vi "Process_data.vi"(3 "No of estimates output":i32=200, 4 "Measurement top level?":bool) -> (6 "Vel stat display":string[][](table), 7 "First Plot data Cluster":cluster{"X array":dbl[], "Y array":dbl[]}[](array[cluster]), 8 "Second Plot Data Cluster":cluster{"X array":dbl[], "Y array":dbl[]}[](array[cluster]))   [LabVIEW 2022 SP3]
uses:
  Controls/Inst_type.ctl
  Controls/Instrument_Array.ctl
  Controls/Post_Process.ctl
  Controls/User_Specific_mode.ctl
  Controls/Server_Comms.ctl
  <vilib>/Analysis/baseanly.llb/Mean (DBL).vi
  Globals/Meas_global.vi
  Globals/Dynamic_call_global.ph.vi
  CTA/CTA Calib Coeff Global.vi
  Globals/LDA_global.vi
  Globals/LDA_meas_global_1.vi
  Acquisition/PWA/PWAtasksGLOBAL.vi
  Globals/Trav_pos_global.vi
  Globals/Preference_global.vi
  <vilib>/Analysis/NI_AALBase.lvlib
panel:
  out "Extra Comments":string
  out "Over/Under string":string
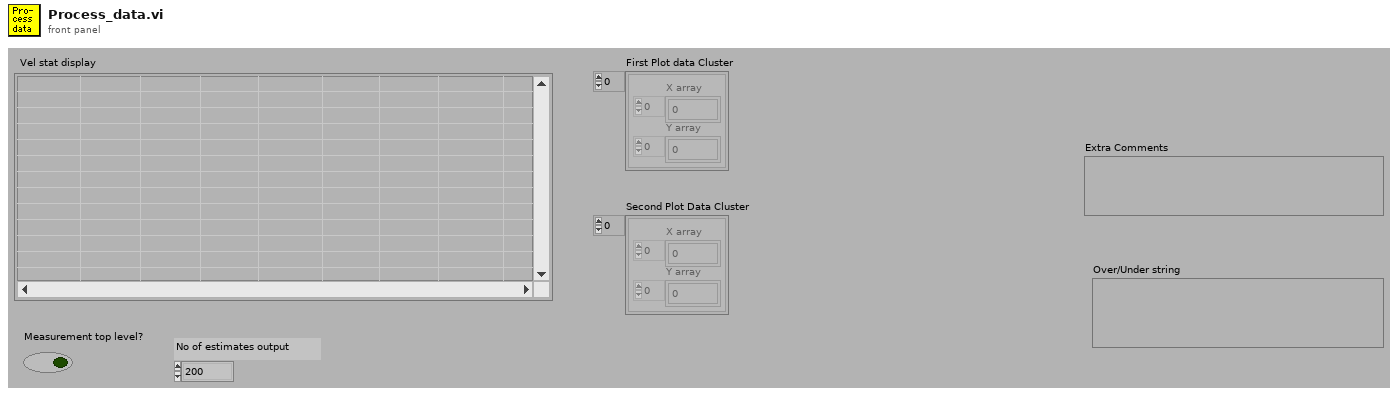
[diagram p1: front panel]
types:
  T1 = typedef "Inst_type.ctl" = enum16{"Raw voltage", "Raw with zero offsetting", "Propeller anemometer", "Pressure Transducer", "Pitot-static tube", "Hot wire", "Cross wire 1", "Cross wire 2", "Generic Linear", "Generic Polynomial", "Generic BackPoly", "Fast FID", "Thermocouple", "Cold wire", "Pulsed Wire", "LDA Vel", "LDA Tran time", "LDA Arr time", "Microphone"}
  T2 = typedef "Instrument_Array.ctl" = enum16{"PWA", "LDA", "Analogue"}
  T3 = enum32{"Invalid", "Standard", "Closed", "Hidden", "Minimized", "Maximized"}
  T4 = typedef "Post_Process.ctl" = enum16{"Take New Data", "Post Process Raw Data File"}
  T5 = typedef "User_Specific_mode.ctl" = enum16{"Check VI only", "Run VI"}
  T6 = enum16{"Save no data", "Save data in new files", "Save data in existing files"}
  T7 = typedef "Server_Comms.ctl" = enum16{"Do Not Link To Server", "Server Link Healthy"}
  T8 = typedef "Analysis_info_cluster.ctl" = cluster{"Colour":u32, "Inst type":T1, "Inst name":string, "Symbol":string, "Code name":string, "Extra Info":string, "Inst Array":T2, "U":dbl, "u^2":dbl, "u^3":dbl, "u^4":dbl, "Skew_u":dbl, "Kurt_u":dbl, "Sd Error in Mean":dbl, "% u'/U":dbl, "X":dbl, "Y":dbl, "Z":dbl, "Timescale integral Estimate":dbl, "Sd Error in Variance":dbl, "Calib File":path, "Calib Constants":dbl[], "Output Position":bool, "Stats":enum16{"None", "Basic", "Full"}, "Av Sampling Rate":dbl, "Av No of Samples":dbl, "Total Meas Time (s)":dbl, "OrigChName":string, "Max value":dbl, "Min value":dbl, "Req Sample Rate Hz":dbl, "Sync Delay Time (s)":dbl, "Ch No":i16, "Device":string, "Use Latest Calib":bool, "Port":string, "Metadata Ch Names":string[], "Metadata Ch Values":string[], "Label":string, "chState":T9, "Point Drift":dbl, "inputConfig":string}
  T9 = typedef "channelState.ctl" = enum32{"No Selection", "Solo", "Mute"}
  T10 = typedef "Time_Trace_Cluster.ctl" = cluster{"Weighting":dbl[], "Voltage":dbl[], "Eng Values":dbl[]}
  T11 = typedef "Calibration data.ctl" = cluster{"X cal.[]":dbl[], "Re cal.[]":dbl[], "a1[]":dbl[], "a2[]":dbl[], "a3[]":dbl[]}
  T12 = typedef "LDA_Channel.ctl" = cluster{"Wavelength (nm)":dbl, "Vel Comp":string, "Max Velocity":dbl, "Min Velocity":dbl, "Max Record length":u16, "Signal gain (dB)":i16, "High voltage":i16, "Optics Conversion Factor":dbl, "Min Record length":u16, "Multiply Velocity by -1":bool, "Signal to Noise Ratio":string, "Validation Ratio":string, "Probe":string, "Laser":string, "BSA":string, "Lense":string, "Beam Separation (mm)":dbl, "Focal Length (mm)":dbl, "COLOUR":u32, "BSA IP":string, "Velocity Range (m/s)":dbl, "Centre Velocity (m/s)":dbl, "Unshifted mW":dbl, "Shifted mW":dbl, "Bandwidth Hz":dbl, "Req Sampling Rate Hz":dbl, "Ch":i32, "CenterFreq Hz":dbl, "Laser IP":string, "Sync Delay (s)":dbl}
  T13 = typedef "PWA_Data.ctl" = enum16{"No PWA Data", "One Ch PWA"}
  T14 = typedef "Resample mode.ctl" = cluster{"Mode":enum16{"Index", "Interpolate"}, "Index":dbl[]}
  T15 = typedef "Shift_Cluster.ctl" = cluster{"Stats":dbl[], "Spectra_Auto":dbl[], "Histogram":dbl[], "Hist Max":dbl, "Hist Min":dbl, "No of Samples":i32, "No in plume":i32, "Weight sum":dbl, "No Of Hist bins":i32, "TimeTrace Max":dbl, "Time Trace Min":dbl, "Trace St Deviation":dbl}
  T16 = typedef "XY_Plot_Cluster.ctl" = cluster{"First Name":string, "Second Name":string, "X axis name":string, "Y axis name":string, "X array":dbl[], "Y array":dbl[], "Weighting":dbl[]}
  T17 = typedef "Traverse_cluster.ctl" = cluster{"Start X":sgl, "Start Y":sgl, "Start Z":sgl, "End X":sgl, "End Y":sgl, "End Z":sgl, "nPoints":i32, "Spacing":T18, "Filename":path, "Tunnel Speed":dbl, "Averaging time (mins)":dbl, "Extra Commands":string, "Carrier_1 Q (l/min)":dbl, "Carrier_2 Q (l/min)":dbl, "Trace Gas Concentration (%)":dbl, "Specific Arguments":string, "Comments":string, "Row No":i32, "Row Type Selector":T19, "EstCompl":string, "Row Duration (mins)":dbl, "nValidPoints":i32, "Meas Setup File":string}
  T18 = typedef "Spacing.ctl" = enum16{"Linear", "Log", "Gauss", "Specified", "N/A"}
  T19 = typedef "Multi_run_mode.ctl" = enum16{"Move Traverse Only", "Set Tunnel Speed Only", "Set Source Only", "Set Measurement Conditions", "Single Measurement", "Vertical Profile", "Lateral Profile", "Longitudinal Profile", "Multi-Axis Profile", "Explore Volume", "Auto Calibrate", "Meas Fast FID Bkgnd", "Check Beam Power", "Scanning Valve Measurement", "Run VI Named:", "Set ADAM Ch", "Wait (minutes)", "Send Message", "Synchronize With:", "Fall Back to this Row", "Turn Off Row Repeating", "Traverse 3D Volume", "Blank Row", "Jump to Fall Back Row"}
  T20 = typedef "Cross_Moments_Shift_Cluster.ctl" = cluster{"Stats":dbl[], "Resampled No of Samples":i32, "Resampled delta T":dbl, "Cross Correlation":dbl[]}
  T21 = typedef "Correlation_cluster1.ctl" = cluster{"U inst":string, "uw":dbl, "u^2w":dbl, "uw^2":dbl, "uw/u'w'":dbl, "W inst":string, "uw^3":dbl, "u^3w":dbl, "u^2w^2":dbl, "Index U":i32, "Index W":i32, "Error info":string[], "Paired Sampling Rate (Hz)":dbl, "u^2 Paired":dbl, "w^2 Paired":dbl, "Time Window (ms)":dbl}
  T22 = typedef "Graph_Type.ctl" = enum16{"Show no graph", "Voltage trace", "Velocity trace", "Vel histogram", "Spectrum", "f.E(f) v Log f", "Auto-Corr"}
  T23 = cluster{"Plot 1":u16, "Plot 2":u16, "Save graph":u16, "Plot Type":T22}
  T24 = cluster{"Plot 1":u16, "Plot 2":u16, "Save graph":u16, "Plot Type":T22}[]
  T25 = typedef "Data for Inst Type.ctl" = enum16{"Eng Values", "Voltage"}
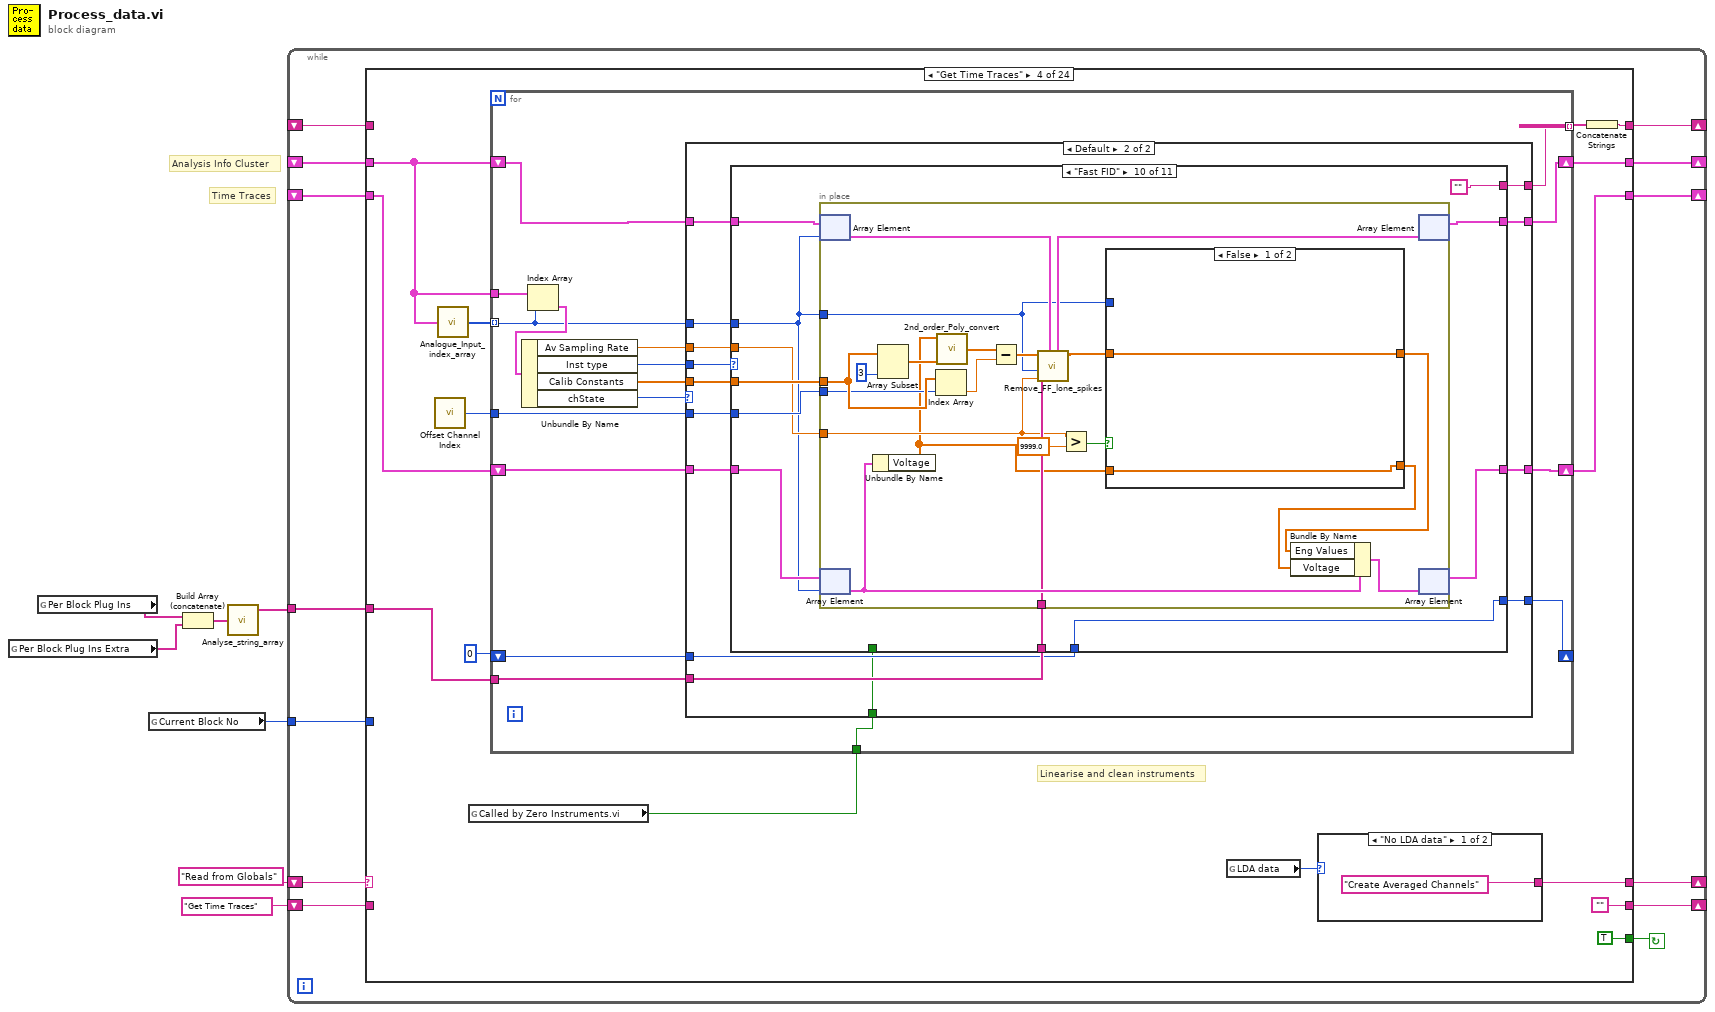
[diagram p0: block diagram]
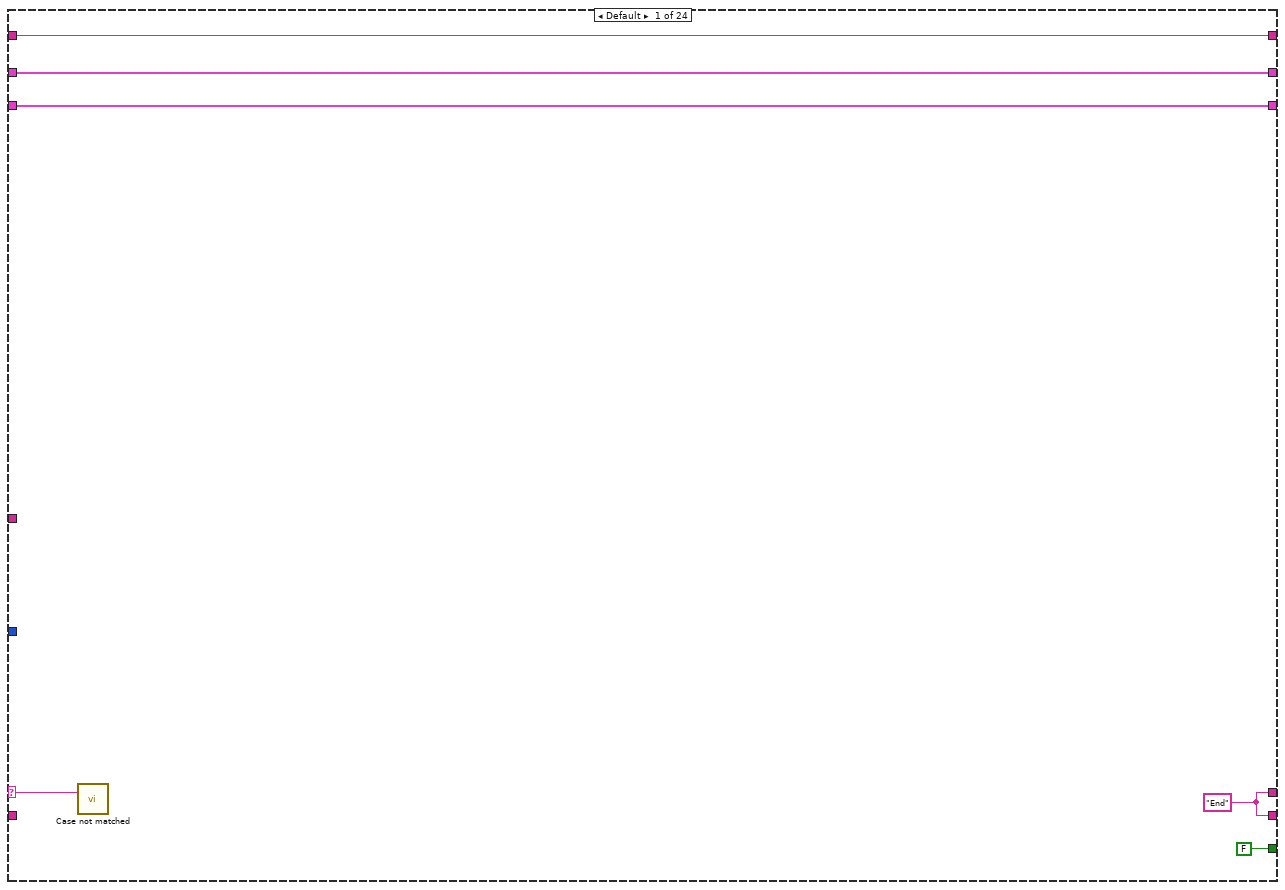
[diagram p2: hidden frame]
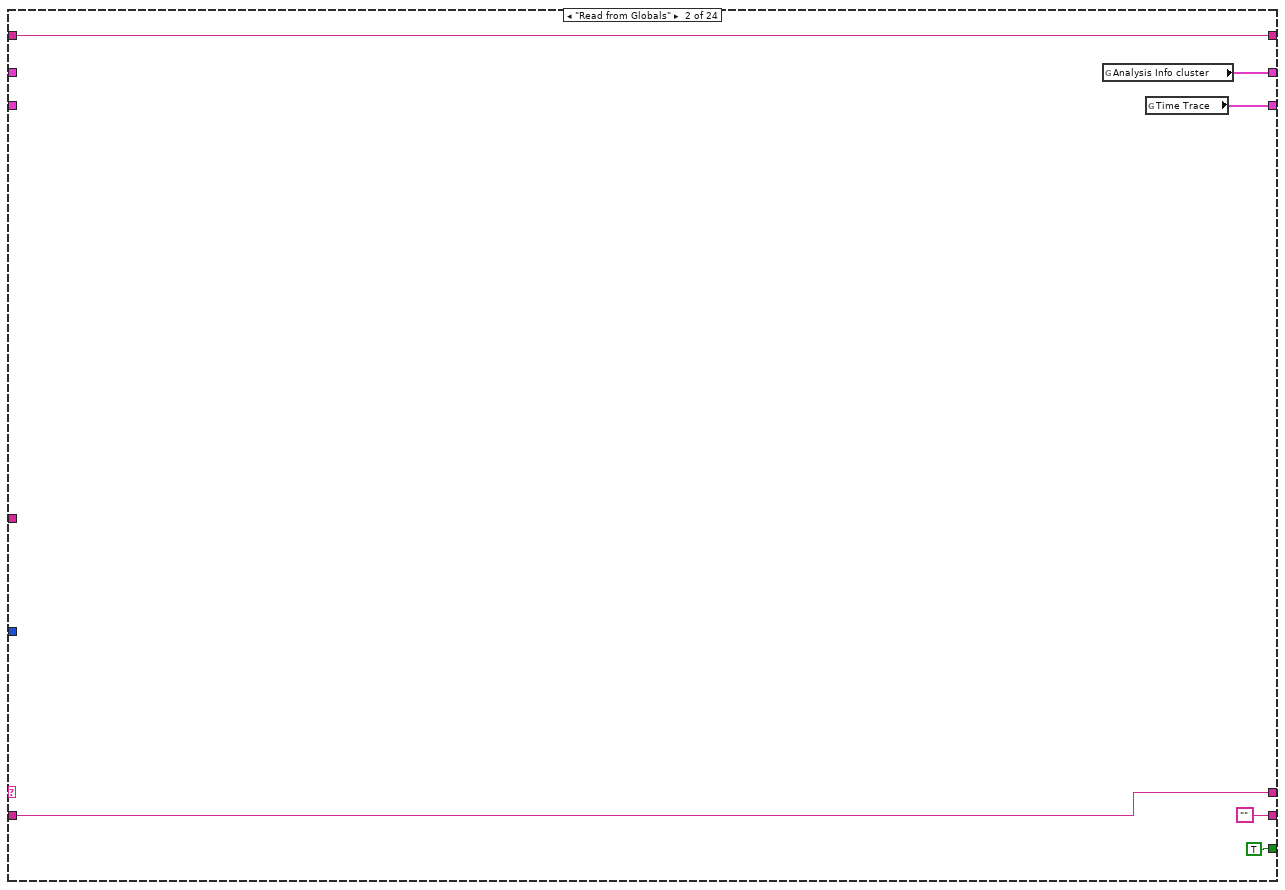
[diagram p3: hidden frame]
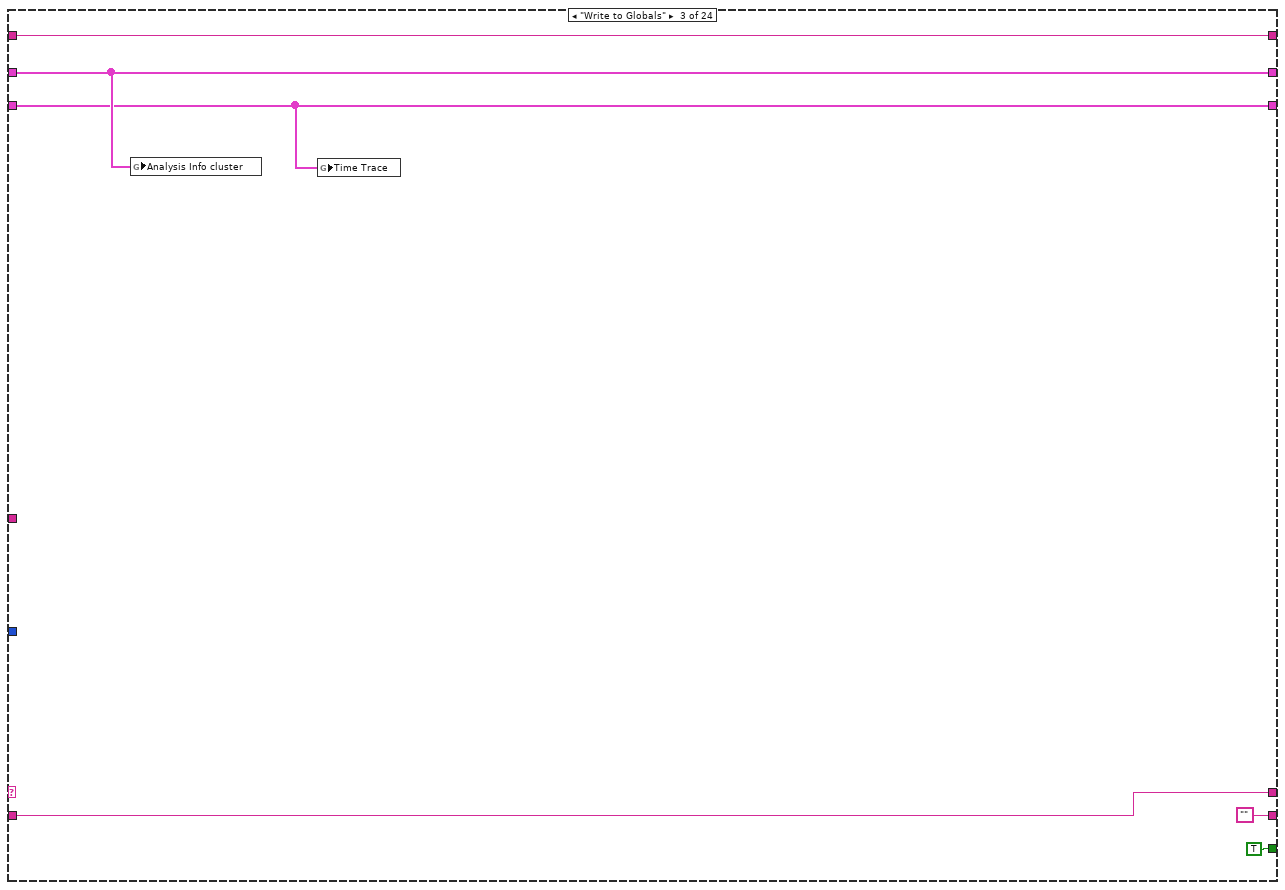
[diagram p4: hidden frame]
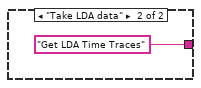
[diagram p5: hidden frame]
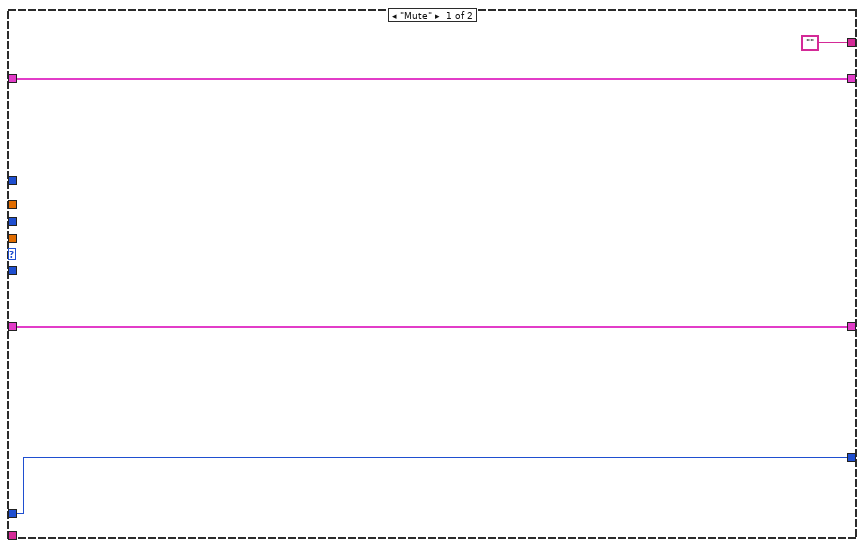
[diagram p6: hidden frame]
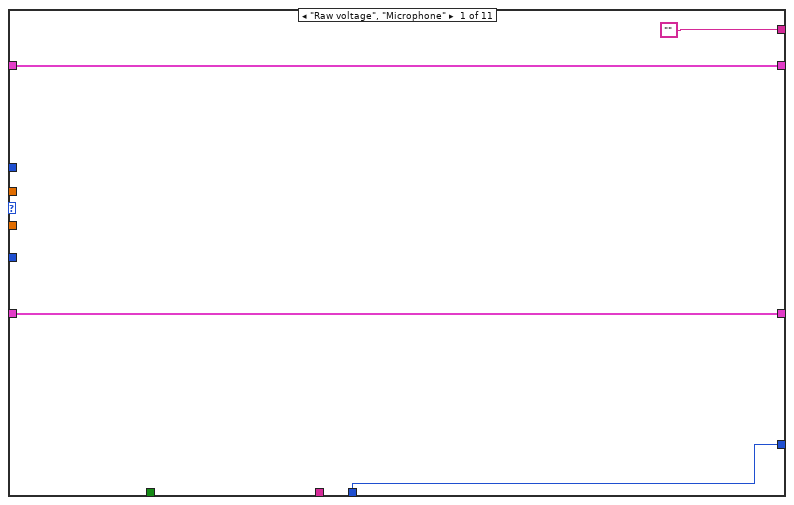
[diagram p7: hidden frame]
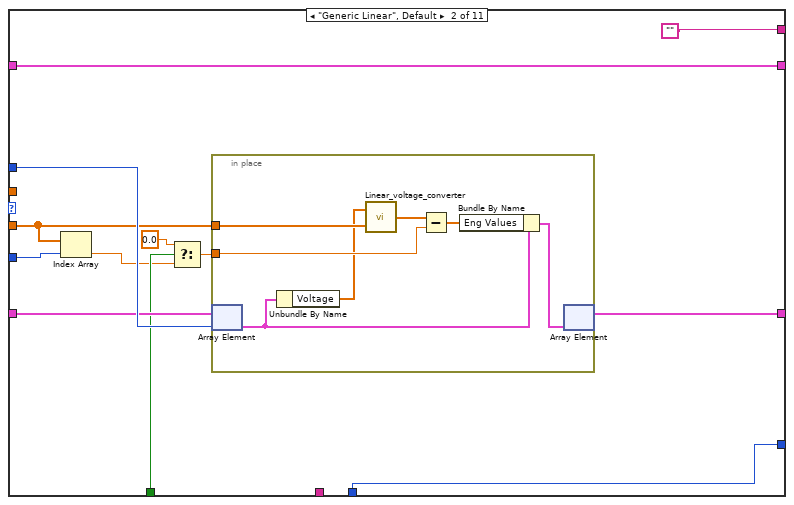
[diagram p8: hidden frame]
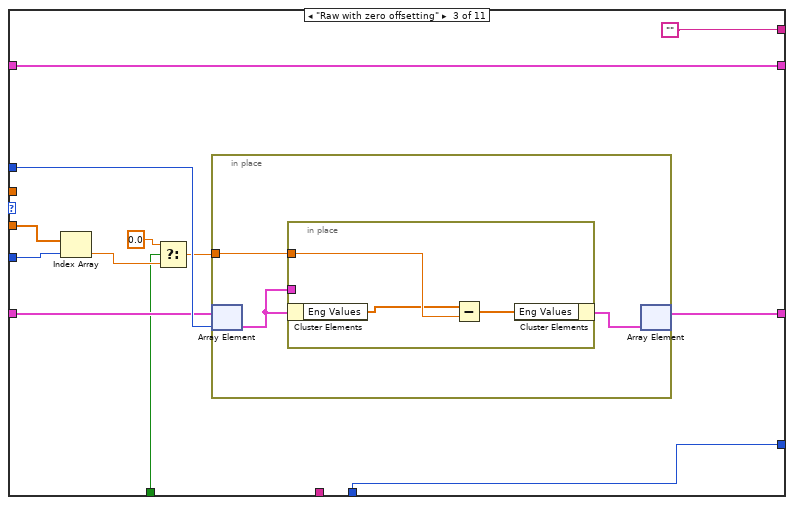
[diagram p9: hidden frame]
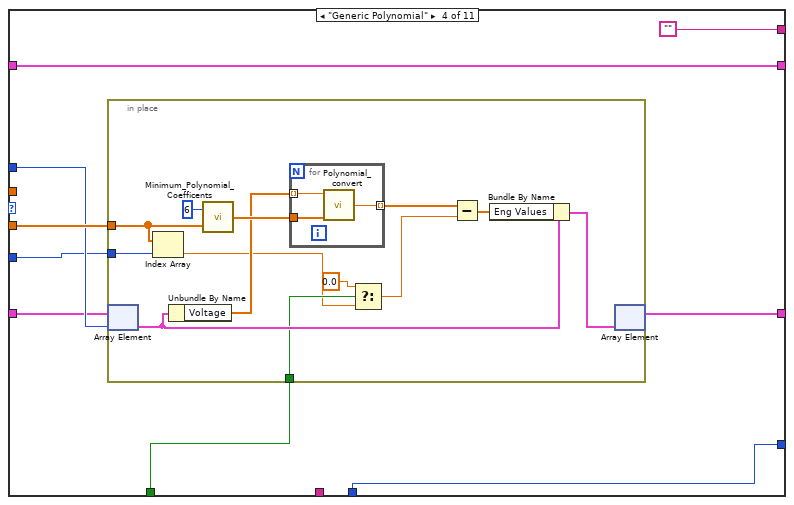
[diagram p10: hidden frame]
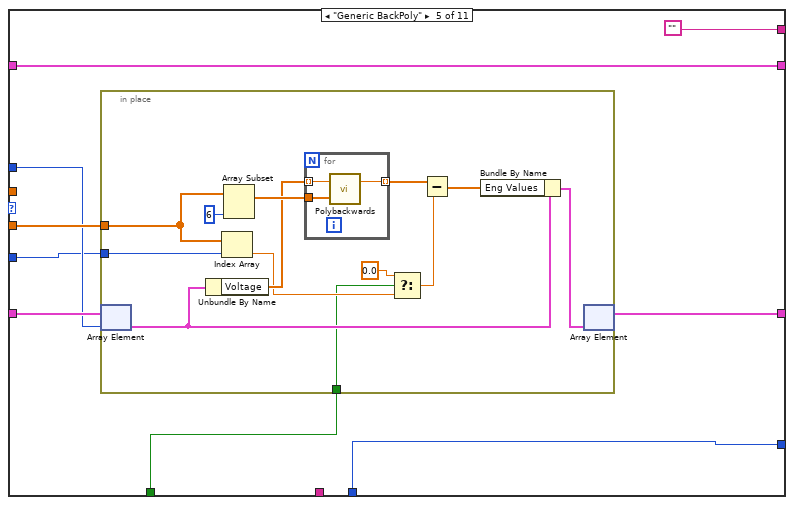
[diagram p11: hidden frame]
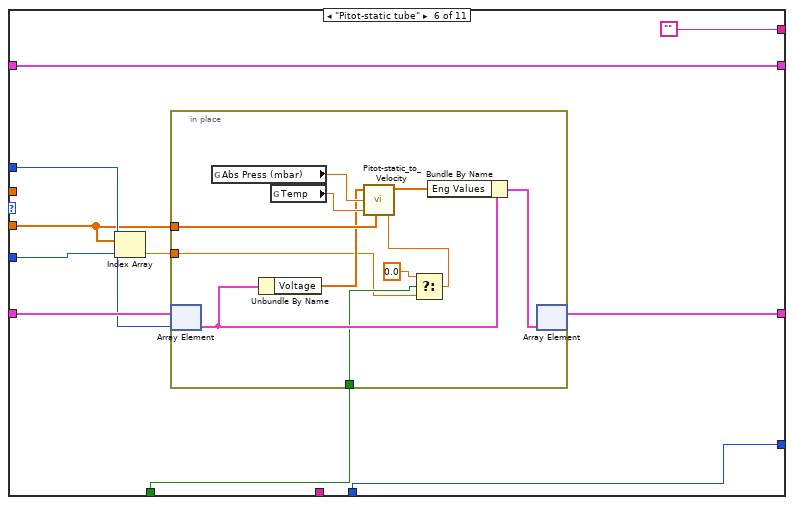
[diagram p12: hidden frame]
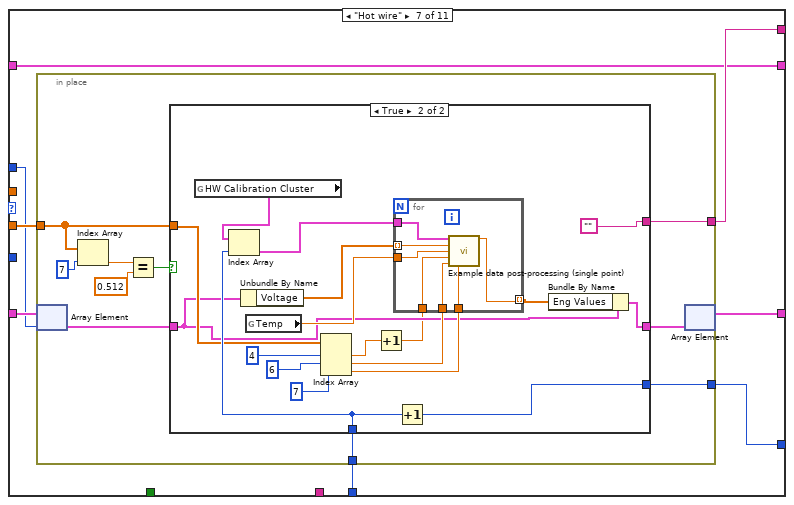
[diagram p13: hidden frame]
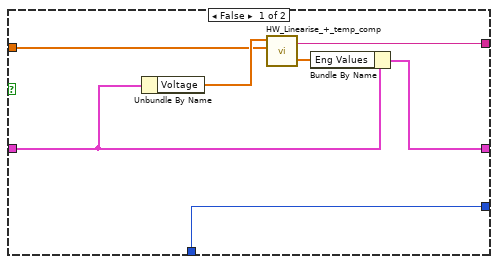
[diagram p14: hidden frame]
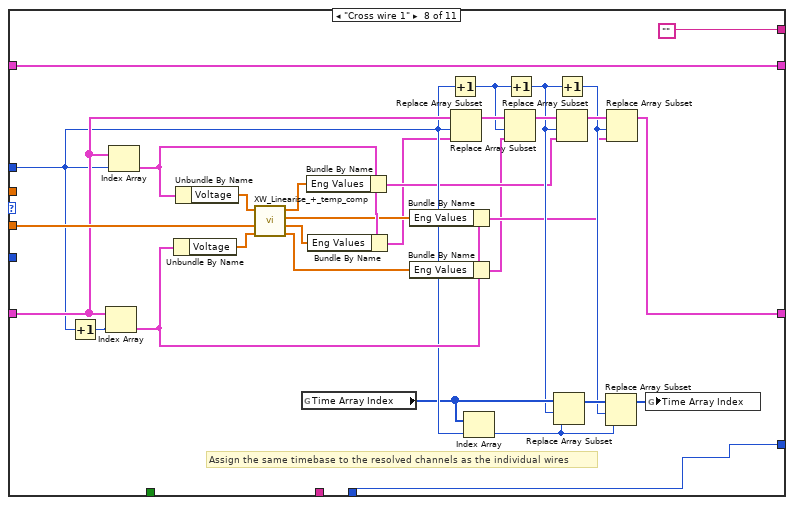
[diagram p15: hidden frame]
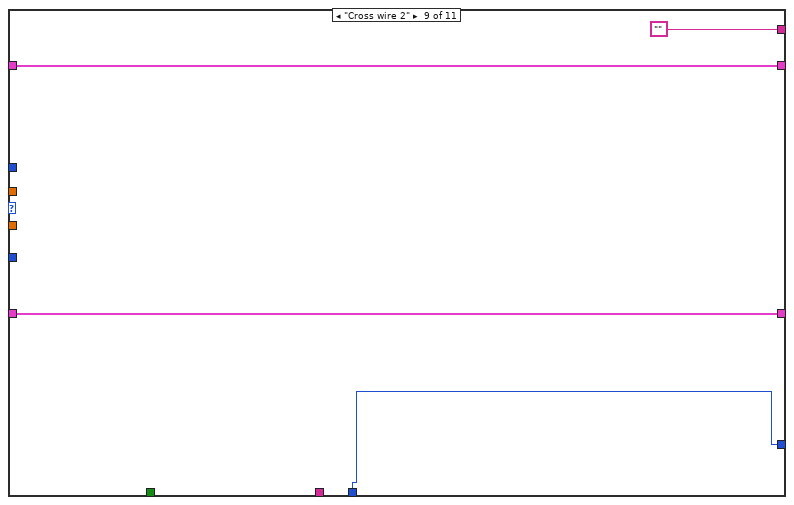
[diagram p16: hidden frame]
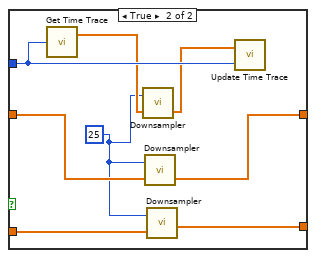
[diagram p17: hidden frame]
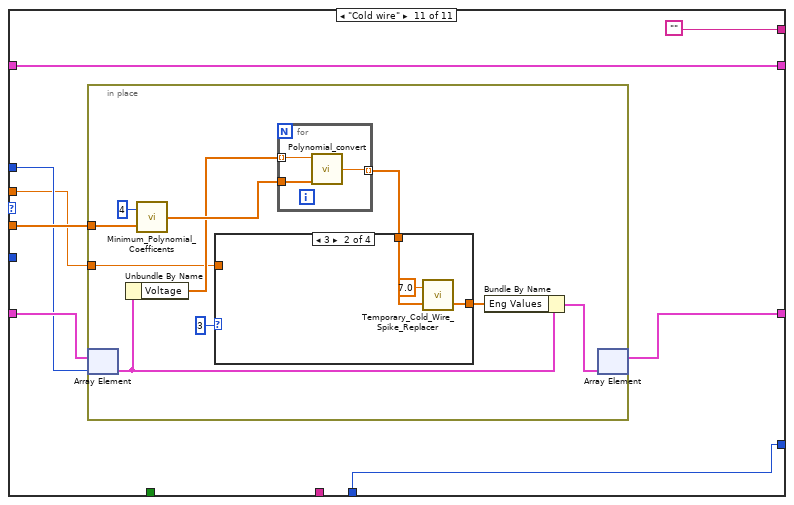
[diagram p18: hidden frame]
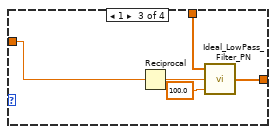
[diagram p20: hidden frame]
diagram:
  # "Time Traces"
  # "Analysis Info Cluster"
  n1 = global read "Dynamic_call_global.ph.vi" "Per Block Plug Ins Extra"() -> (w4:string[])
  n2 = global read "Dynamic_call_global.ph.vi" "Per Block Plug Ins"() -> (w3:string[])
  n3 = global read "Meas_global.vi" "Current Block No"() -> (w6:i32)
  n4 = Build Array (concatenate)(w3, w4) -> (w2:string[])
  n5 = call "Analyse_string_array.vi"("String array"=w2) -> ("Unique strings"=w1:string[])  [unwired: 2 out]
  n6 = while {
    shift-right: [w19] -> _
    shift-left: "Read from Globals" -> [w20]
    shift-right: [w17] -> _
    shift-left: _ -> [w18]
    shift-right: [w13] -> _
    shift-left: _ -> [w12]
    shift-right: [w16] -> _
    shift-left: _ -> [w14]
    tunnel: w6 -> [w11]
    shift-right: [w9] -> _
    shift-left: "Get Time Traces" -> [w10]
    tunnel: w1 -> [w8]
    stop <- w15 continue-if-true
    n7 = case shown="\"Get Time Traces\"" w20 {
      selector: w20 -> [w26 _ _ _ _ _ _ _ _ _ _ _ _ _ _ _ _ _ _ _ _ _ _ _]
      tunnel: [w21 w29 w37 w50 w363 "LDA_Angular_Alignment_Tweak" w507 "Any Pre Analysis Plugins?" w672 "Read from Globals" "Add Extra Data Channels" "Min Max Limiter" "Analysis of Time Traces" "Vel Stats Display" w920 "Write to Globals" "Write to Globals" w1162 w1174 "Output Cross moments" "Create Plot Clusters" "Seeder Control?" "Control Seeding level" "End"] -> w19
      tunnel: w12 -> [w23 _ w34 w44 w374 w442 w506 w607 w674 w690 w719 w821 w885 w912 w923 w1012 w1063 w1160 w1179 w1337 w1387 w1418 w1520 w1536]
      tunnel: w18 -> [w22 _ w33 w49 w377 w441 w523 w610 w673 w689 w718 w822 w888 w911 w922 w1013 w1067 w1164 w1176 w1336 w1386 w1420 w1519 w1534]
      tunnel: [w22 w31 w33 w48 w376 w441 w522 w605 w673 w689 w718 w823 w887 w911 w922 w1013 w1067 w1164 w1177 w1336 w1386 w1420 w1519 w1534] -> w17
      tunnel: [w24 w30 w38 w47 w378 w443 w521 w613 w675 w691 w720 w820 w886 w916 w924 w1011 w1068 w1165 w1181 w1354 w1388 w1425 w1521 w1535] -> w16
      tunnel: [FALSE TRUE TRUE TRUE TRUE TRUE TRUE TRUE TRUE TRUE TRUE TRUE TRUE TRUE TRUE TRUE TRUE TRUE w1173 TRUE TRUE w1426 w1531 FALSE] -> w15
      tunnel: w14 -> [w24 w30 w38 _ w379 w443 w521 w613 w675 w691 w720 w820 w886 w917 w924 w1011 w1068 w1165 w1180 w1354 w1388 w1425 w1521 w1535]
      tunnel: [w23 w32 w34 w43 w375 w442 w506 w607 w674 w690 w719 w821 w885 w905 w923 w1012 w1064 w1160 w1178 w1337 w1387 w1418 w1520 w1536] -> w13
      tunnel: w11 -> [_ _ _ _ w373 _ _ _ _ _ w715 _ _ _ _ _ _ _ w1175 _ _ _ _ _]
      tunnel: w10 -> [_ w29 w37 _ _ _ w514 _ _ _ _ _ _ _ _ _ _ _ _ _ _ _ _ _]
      tunnel: [w21 "" "" "" "" "1" w511 "" w671 "Add PWA Data" "" "" "" "" "" "Per Block Plug ins" "Per Block Plug ins" w1161 w1172 "" "" "" "" ""] -> w9
      tunnel: w8 -> [_ _ _ w41 _ _ _ _ _ _ _ _ _ _ _ _ _ w1159 _ _ _ _ _ _]
      frame Default {
        w21 = "End"
        n8 = call "Case not matched.vi"("Case Name not Matched"=w26) -> ()
      }
      frame "Read from Globals" {
        n9 = global read "Meas_global.vi" "Analysis Info cluster"() -> (w32:T8[])
        n10 = global read "Meas_global.vi" "Time Trace"() -> (w31:T10[])
      }
      frame "Write to Globals" {
        n11 = global write "Meas_global.vi" "Analysis Info cluster"(w34) -> ()
        n12 = global write "Meas_global.vi" "Time Trace"(w33) -> ()
      }
      frame "Get Time Traces" {
        # "Linearise and clean instruments"
        n13 = call "Offset Channel Index.vi"() -> ("index"=w42:i32)
        n14 = call "Analogue_Input_index_array.vi"("Analysis Info cluster"=w44) -> ("Array"=w53:i32[])
        n15 = global read "Meas_global.vi" "Called by Zero Instruments.vi"() -> (w39:bool)
        n16 = for {
          shift-right: [w69] -> w48
          shift-left: w49 -> [w70]
          tunnel: w44 -> [w72]
          tunnel: w53 -> [w66] mode=indexing
          tunnel: [w64] -> w52 mode=indexing
          shift-right: [w62] -> w43
          shift-left: w44 -> [w63]
          tunnel: w42 -> [w61]
          tunnel: w41 -> [w60]
          shift-right: [w58] -> _
          shift-left: 0 -> [w59]
          tunnel: w39 -> [w57]
          n17 = Index Array(array=w72, index=w66) -> (element=w71:T8)
          n18 = Unbundle By Name(w71) -> ("Av Sampling Rate"=w65:dbl, "Inst type"=w68:T1, "Calib Constants"=w67:dbl[], "chState"=w56:T9)
          n19 = case shown="Default" w56 {
            tunnel: w70 -> [w74 w90]
            tunnel: [w74 w89] -> w69
            tunnel: w68 -> [_ w88]
            tunnel: w67 -> [_ w87]
            tunnel: w66 -> [_ w86]
            tunnel: w65 -> [_ w85]
            tunnel: ["" w84] -> w64
            tunnel: w63 -> [w76 w83]
            tunnel: [w76 w82] -> w62
            tunnel: w61 -> [_ w81]
            tunnel: w60 -> [_ w80]
            tunnel: w59 -> [w73 w79]
            tunnel: [w73 w78] -> w58
            tunnel: w57 -> [_ w77]
            frame "Mute" {
            }
            frame Default {
              n20 = case shown="\"Fast FID\"" w88 {
                tunnel: w87 -> [_ w103 w122 w140 w165 w188 w210 w282 _ w297 w335]
                tunnel: w86 -> [_ w106 w125 w139 w163 w190 w207 w264 _ w288 w332]
                tunnel: w90 -> [w92 w105 w124 w138 w164 w191 w209 w276 w286 w296 w334]
                tunnel: [w92 w104 w123 w137 w162 w189 w208 w274 w286 w295 w333] -> w89
                tunnel: w81 -> [_ w102 w121 w136 w161 w187 _ _ _ w294 _]
                tunnel: w85 -> [_ _ _ _ _ _ _ _ _ w293 w331]
                tunnel: ["" "" "" "" "" "" w206 "" "" "" ""] -> w84
                tunnel: w83 -> [w93 w100 w119 w134 w159 w184 w205 w270 w284 w291 w329]
                tunnel: [w93 w100 w119 w134 w159 w184 w205 w270 w284 w290 w329] -> w82
                tunnel: w80 -> [_ _ _ _ _ _ _ _ _ w289 _]
                tunnel: w79 -> [w91 w99 w118 w133 w158 w183 w204 w253 w283 w287 w328]
                tunnel: [w91 w99 w118 w133 w158 w183 w203 w253 w283 w287 w328] -> w78
                tunnel: w77 -> [_ w98 w115 w132 w157 w182 _ _ _ _ _]
                frame "Raw voltage", "Microphone" {
                }
                frame "Generic Linear", Default {
                  n21 = Index Array(array=w103, index=w102) -> (element=w97:dbl)
                  n22 = Select(t=0.0, s=w98, f=w97) -> (s? t:f=w95:dbl)
                  n23 = in-place {
                    in-place-border: w103 -> [w113]
                    in-place-border: w95 -> [w109]
                    n24 = in-place-array #1(w105, w106) -> (w108:T10)
                    n25 = Unbundle By Name(w108) -> ("Voltage"=w107:dbl[])
                    n26 = call "Linear_voltage_converter.vi"("Caib const A,B"=w113, "Voltage array"=w107) -> ("Converted array"=w111:dbl[])
                    n27 = Subtract(x=w111, y=w109) -> (x-y=w110:dbl[])
                    n28 = Bundle By Name(cluster=w108, "Eng Values"=w110) -> (w112:T10)
                    n29 = in-place-array #1(w112) -> (w104:T10[])  [unwired: 1 out]
                  }
                }
                frame "Raw with zero offsetting" {
                  n30 = Index Array(array=w122, index=w121) -> (element=w116:dbl)
                  n31 = Select(t=0.0, s=w115, f=w116) -> (s? t:f=w114:dbl)
                  n32 = in-place {
                    in-place-border: w114 -> [w128]
                    n33 = in-place-array #2(w124, w125) -> (w127:T10)
                    n34 = in-place {
                      in-place-border: w128 -> [w131]
                      in-place-border: w127 -> [_]
                      n35 = in-place-cluster #3(w127) -> ("Eng Values"=w129:dbl[])
                      n36 = Subtract(x=w129, y=w131) -> (x-y=w130:dbl[])
                      n37 = in-place-cluster #3("Eng Values"=w130) -> (w126:T10)
                    }
                    n38 = in-place-array #2(w126) -> (w123:T10[])  [unwired: 1 out]
                  }
                }
                frame "Generic Polynomial" {
                  n39 = in-place {
                    in-place-border: w140 -> [w148]
                    in-place-border: w136 -> [w147]
                    in-place-border: w132 -> [w143]
                    n40 = in-place-array #4(w138, w139) -> (w146:T10)
                    n41 = Index Array(array=w148, index=w147) -> (element=w142:dbl)
                    n42 = Unbundle By Name(w146) -> ("Voltage"=w145:dbl[])
                    n43 = call "Minimum_Polynomial_Coefficents.vi"("Calib consts"=w148, "Max Length"=6) -> ("Coefficients"=w152:dbl[])
                    n44 = for {
                      tunnel: w152 -> [w156]
                      tunnel: w145 -> [w155] mode=indexing
                      tunnel: [w154] -> w150 mode=indexing
                      n45 = call "Polynomial_convert.vi"("Calib constants"=w156, "Voltage"=w155) -> ("Eng Values"=w154:dbl)  [unwired: 4 out]
                    }
                    n46 = Select(t=0.0, s=w143, f=w142) -> (s? t:f=w141:dbl)
                    n47 = Subtract(x=w150, y=w141) -> (x-y=w149:dbl[])
                    n48 = Bundle By Name(cluster=w146, "Eng Values"=w149) -> (w151:T10)
                    n49 = in-place-array #4(w151) -> (w137:T10[])  [unwired: 1 out]
                  }
                }
                frame "Generic BackPoly" {
                  n50 = in-place {
                    in-place-border: w165 -> [w175]
                    in-place-border: w161 -> [w174]
                    in-place-border: w157 -> [w166]
                    n51 = in-place-array #5(w164, w163) -> (w171:T10)
                    n52 = Unbundle By Name(w171) -> ("Voltage"=w170:dbl[])
                    n53 = Index Array(array=w175, index=w174) -> (element=w168:dbl)
                    n54 = Array Subset(array=w175, length=6) -> (w178:dbl[])  [unwired: 1 in]
                    n55 = for {
                      tunnel: w178 -> [w181]
                      tunnel: w170 -> [w180] mode=indexing
                      tunnel: [w179] -> w173 mode=indexing
                      n56 = call "Polybackwards.vi"("Coefficients"=w181, "Y input"=w180) -> ("X output"=w179:dbl)  [unwired: 1 out]
                    }
                    n57 = Select(t=0.0, s=w166, f=w168) -> (s? t:f=w167:dbl)
                    n58 = Subtract(x=w173, y=w167) -> (x-y=w172:dbl[])
                    n59 = Bundle By Name(cluster=w171, "Eng Values"=w172) -> (w176:T10)
                    n60 = in-place-array #5(w176) -> (w162:T10[])  [unwired: 1 out]
                  }
                }
                frame "Pitot-static tube" {
                  n61 = Index Array(array=w188, index=w187) -> (element=w186:dbl)
                  n62 = in-place {
                    in-place-border: w188 -> [w202]
                    in-place-border: w186 -> [w193]
                    in-place-border: w182 -> [w194]
                    n63 = in-place-array #6(w191, w190) -> (w197:T10)
                    n64 = global read "Meas_global.vi" "Abs Press (mbar)"() -> (w201:dbl)
                    n65 = Unbundle By Name(w197) -> ("Voltage"=w196:dbl[])
                    n66 = global read "Meas_global.vi" "Temp"() -> (w198:dbl)
                    n67 = Select(t=0.0, s=w194, f=w193) -> (s? t:f=w192:dbl)
                    n68 = call "Pitot-static_to_Velocity.vi"("Pressure Trans voltage"=w196, "Atmos Press mbar  (1000)"=w201, "Temp  C  (20)"=w198, "Pressure Trans Calib const"=w202, "Mano Zero"=w192) -> ("Velocity (m/s)"=w200:dbl[])  [unwired: 1 in, 2 out]
                    n69 = Bundle By Name(cluster=w197, "Eng Values"=w200) -> (w199:T10)
                    n70 = in-place-array #6(w199) -> (w189:T10[])  [unwired: 1 out]
                  }
                }
                frame "Hot wire" {
                  n71 = in-place {
                    in-place-border: w210 -> [w216]
                    in-place-border: [w218] -> w206
                    in-place-border: w204 -> [w215]
                    in-place-border: [w214] -> w203
                    n72 = in-place-array #7(w209, w207) -> (w219:T10)
                    n73 = Index Array(array=w216, index=7) -> (element=w213:dbl)
                    n74 = Equal?(x=w213, y=0.512) -> (x = y?=w212:bool)
                    n75 = case shown="True" w212 {
                      tunnel: [w226 w230] -> w220
                      tunnel: w219 -> [w225 w231]
                      tunnel: [w224 ""] -> w218
                      tunnel: w216 -> [w222 w239]
                      tunnel: w215 -> [w221 w244]
                      tunnel: [w221 w243] -> w214
                      frame False {
                        n76 = Unbundle By Name(w225) -> ("Voltage"=w223:dbl[])
                        n77 = call "HW_Linearise_+_temp_comp.vi"("Caib const"=w222, "HW voltage"=w223) -> ("Velocity"=w227:dbl[], "Error string"=w224:string)  [unwired: 4 in]
                        n78 = Bundle By Name(cluster=w225, "Eng Values"=w227) -> (w226:T10)
                      }
                      frame True {
                        n79 = global read "CTA Calib Coeff Global.vi" "HW Calibration Cluster"() -> (w245:T11[])
                        n80 = Index Array(array=w245, index=w244) -> (element=w242:T11)
                        n81 = Unbundle By Name(w231) -> ("Voltage"=w241:dbl[])
                        n82 = global read "Meas_global.vi" "Temp"() -> (w240:dbl)
                        n83 = Index Array(array=w239, index #1=4 ("index"), index #2=6 ("index"), index #3=7 ("index")) -> (element #1=w238:dbl, element #2=w237:dbl, element #3=w236:dbl)
                        n84 = Increment(x=w238) -> (x+1=w228:dbl)
                        n85 = for {
                          tunnel: w242 -> [w252]
                          tunnel: w241 -> [w251] mode=indexing
                          tunnel: w240 -> [w250]
                          tunnel: w228 -> [w249]
                          tunnel: w237 -> [w248]
                          tunnel: w236 -> [w247]
                          tunnel: [w246] -> w232 mode=indexing
                          n86 = call "Example data post-processing (single point).vi"("Calibration data"=w252, "V_out (V)"=w251, "Ta (°C)"=w250, "Overheat ratio (Rw / R0)"=w249, "Gain"=w248, "Offset (V)"=w247) -> ("U (m/s)"=w246:dbl)  [unwired: 9 in]
                        }
                        n87 = Increment(x=w244) -> (x+1=w243:i32)
                        n88 = Bundle By Name(cluster=w231, "Eng Values"=w232) -> (w230:T10)
                      }
                    }
                    n89 = in-place-array #7(w220) -> (w208:T10[])  [unwired: 1 out]
                  }
                }
                frame "Cross wire 1" {
                  # "Assign the same timebase to the resolved channels as the individual wires"
                  n90 = Increment(x=w264) -> (x+1=w279:i32)
                  n91 = Index Array(array=w276, index=w279) -> (element=w277:T10)
                  n92 = Index Array(array=w276, index=w264) -> (element=w278:T10)
                  n93 = Unbundle By Name(w277) -> ("Voltage"=w281:dbl[])
                  n94 = Unbundle By Name(w278) -> ("Voltage"=w280:dbl[])
                  n95 = call "XW_Linearise_+_temp_comp.vi"("XW2 voltage"=w281, "Calib const"=w282, "XW1 voltage"=w280) -> ("V"=w265:dbl[], "U"=w266:dbl[], "U2"=w267:dbl[], "U1"=w268:dbl[])  [unwired: 5 in]
                  n96 = global read "Meas_global.vi" "Time Array Index"() -> (w263:i32[])
                  n97 = Bundle By Name(cluster=w278, "Eng Values"=w268) -> (w257:T10)
                  n98 = Bundle By Name(cluster=w278, "Eng Values"=w266) -> (w256:T10)
                  n99 = Bundle By Name(cluster=w277, "Eng Values"=w267) -> (w255:T10)
                  n100 = Bundle By Name(cluster=w277, "Eng Values"=w265) -> (w254:T10)
                  n101 = Increment(x=w264) -> (x+1=w269:i32)
                  n102 = Replace Array Subset(array=w276, new element=w256, index=w264) -> (w275:T10[])
                  n103 = Index Array(array=w263, index=w264) -> (element=w259:i32)
                  n104 = Replace Array Subset(array=w275, new element=w254, index=w269) -> (w273:T10[])
                  n105 = Increment(x=w269) -> (x+1=w262:i32)
                  n106 = Replace Array Subset(array=w263, new element=w259, index=w262) -> (w261:i32[])
                  n107 = Increment(x=w262) -> (x+1=w260:i32)
                  n108 = Replace Array Subset(array=w273, new element=w257, index=w262) -> (w272:T10[])
                  n109 = Replace Array Subset(array=w261, new element=w259, index=w260) -> (w258:i32[])
                  n110 = Replace Array Subset(array=w272, new element=w255, index=w260) -> (w274:T10[])
                  n111 = global write "Meas_global.vi" "Time Array Index"(w258) -> ()
                }
                frame "Cross wire 2" {
                }
                frame "Fast FID" {
                  n112 = in-place {
                    in-place-border: w297 -> [w314]
                    in-place-border: w294 -> [w310]
                    in-place-border: w293 -> [w302]
                    in-place-border: w289 -> [w306]
                    in-place-border: w288 -> [w303]
                    n113 = in-place-array #8(w291, w288) -> (w308:T8)
                    n114 = in-place-array #9(w296, w288) -> (w309:T10)
                    n115 = Unbundle By Name(w309) -> ("Voltage"=w299:dbl[])
                    n116 = Array Subset(array=w314, length=3) -> (w313:dbl[])  [unwired: 1 in]
                    n117 = Index Array(array=w314, index=w310) -> (element=w317:dbl)
                    n118 = call "2nd_order_Poly_convert.vi"("Calib constants"=w313, "Voltage"=w299) -> ("Eng Values"=w312:dbl[])  [unwired: 4 out]
                    n119 = Subtract(x=w312, y=w317) -> (x-y=w316:dbl[])
                    n120 = call "Remove_FF_lone_spikes.vi"("Analysis Info cluster In"=w308, "Average Sampling Rate"=w302, "index of element"=w303, "Per Block Plug Ins"=w306, "Time Trace"=w316) -> ("Filtered Time Trace"=w304:dbl[], "Analysis Info cluster Out"=w307:T8)  [unwired: 3 in]
                    n121 = Greater?(x=w302, y=9999.0) -> (0:w300:bool)
                    n122 = case shown="False" w300 {
                      tunnel: [w319 w327] -> w305
                      tunnel: w304 -> [w319 w326]
                      tunnel: w303 -> [_ w325]
                      tunnel: w299 -> [w318 w321]
                      tunnel: [w318 w320] -> w298
                      frame False {
                      }
                      frame True {
                        w322 = 25 ("Averaging samples")
                        n123 = call "Get Time Trace.vi"("Channel Index"=w325) -> ("Time (s)"=w324:dbl[])  [unwired: 1 out]
                        n124 = call "Downsampler.vi"("Input Array"=w324, "Averaging samples"=w322) -> ("Downsampled Array"=w323:dbl[])  [unwired: 1 out]
                        n125 = call "Downsampler.vi"("Input Array"=w326, "Averaging samples"=w322) -> ("Downsampled Array"=w327:dbl[])  [unwired: 1 out]
                        n126 = call "Downsampler.vi"("Input Array"=w321, "Averaging samples"=w322) -> ("Downsampled Array"=w320:dbl[])  [unwired: 1 out]
                        n127 = call "Update Time Trace.vi"("Channel Index"=w325, "Time (s)"=w323) -> ()  [unwired: 1 in]
                      }
                    }
                    n128 = Bundle By Name(cluster=w309, "Eng Values"=w305, "Voltage"=w298) -> (w311:T10)
                    n129 = in-place-array #8(w307) -> (w290:T8[])  [unwired: 1 out]
                    n130 = in-place-array #9(w311) -> (w295:T10[])  [unwired: 1 out]
                  }
                }
                frame "Cold wire" {
                  n131 = in-place {
                    in-place-border: w335 -> [w344]
                    in-place-border: w331 -> [w336]
                    n132 = in-place-array #10(w334, w332) -> (w338:T10)
                    n133 = Unbundle By Name(w338) -> ("Voltage"=w337:dbl[])
                    n134 = call "Minimum_Polynomial_Coefficents.vi"("Calib consts"=w344, "Max Length"=4) -> ("Coefficients"=w343:dbl[])
                    n135 = for {
                      tunnel: w343 -> [w362]
                      tunnel: w337 -> [w361] mode=indexing
                      tunnel: [w360] -> w342 mode=indexing
                      n136 = call "Polynomial_convert.vi"("Calib constants"=w362, "Voltage"=w361) -> ("Eng Values"=w360:dbl)  [unwired: 4 out]
                    }
                    n137 = case shown="3" 3 {
                      tunnel: w342 -> [w346 w349 w353 w358]
                      tunnel: [w346 w348 w351 w357] -> w340
                      tunnel: w336 -> [_ _ w350 w355]
                      frame 0, Default {
                      }
                      frame 3 {
                        n138 = call "Temporary_Cold_Wire_Spike_Replacer.vi"("Data in"=w349, "St Dev threshold"=7.0) -> ("Data out"=w348:dbl[])  [unwired: 1 out]
                      }
                      frame 1 {
                        n139 = Reciprocal(x=w350) -> (1/x=w354:dbl)
                        n140 = call "Ideal_LowPass_Filter_PN.vi"("Cutoff frequency (Hz)"=100.0, "dt (s)"=w354, "1D Data (uniform spacing)"=w353) -> ("Low-pass filtered 1D Data"=w351:dbl[])
                      }
                      frame 2 {
                        n141 = Reciprocal(x=w355) -> (1/x=w359:dbl)
                        n142 = call "Ideal_Notch_Filter_PN.vi"("Frequencies to cut (Hz)"=dbl[] [150.0, 250.0], "dt (s)"=w359, "1D Data (uniform spacing)"=w358) -> ("Low-pass filtered 1D Data"=w357:dbl[])
                      }
                    }
                    n143 = Bundle By Name(cluster=w338, "Eng Values"=w340) -> (w339:T10)
                    n144 = in-place-array #10(w339) -> (w333:T10[])  [unwired: 1 out]
                  }
                }
              }
            }
          }
        }
        n145 = global read "Meas_global.vi" "LDA data"() -> (w51:enum16{"No LDA data", "Take LDA data"})
        n146 = case shown="\"No LDA data\"" w51 {
          tunnel: ["Create Averaged Channels" "Get LDA Time Traces"] -> w50
          frame "No LDA data" {
          }
          frame "Take LDA data" {
          }
        }
        n147 = Concatenate Strings(w52) -> (w47:string)
      }
      frame "Get LDA Time Traces" {
        w367 = 3083254242.0  # 13/9/01 When new synchronisation routine was implemented
        n148 = global read "LDA_global.vi" "Non-coincident"() -> (w371:bool)
        n149 = global read "Meas_global.vi" "Use  Analogue channel to software sync with LDA"() -> (w370:bool)
        n150 = global read "Meas_global.vi" "Time Data was Aquired"() -> (w368:dbl)
        n151 = Greater?(x=w368, y=w367) -> (0:w369:bool)
        n152 = Compound Arithmetic op=AND(w370, w369) -> (w365:bool)
        n153 = case shown="True" w371 {
          tunnel: w379 -> [w387 w392]
          tunnel: [w386 w392] -> w378
          tunnel: w377 -> [w384 w395]
          tunnel: [w383 w394] -> w376
          tunnel: [w381 w393] -> w375
          tunnel: w374 -> [w382 w390]
          tunnel: w373 -> [_ w391]
          tunnel: w365 -> [w385 _]
          frame False {
            n154 = Not(x=w385) -> (.not. x?=w389:bool)
            n155 = call "LDA_High_Convert_New.vi"("Analysis Info cluster"=w382, "Create Sync Index"=w389, "Time Trace in"=w384) -> ("Analysis Info cluster Out"=w381:T8[], "Error String"=w388:string, "Time Trace out"=w383:T10[])  [unwired: 2 in, 2 out]
            n156 = Concatenate Strings(w387, w388) -> (w386:string)
          }
          frame True {
            n157 = global read "LDA_global.vi" "LDA Channels"() -> (w396:T12[])
            n158 = global read "LDA_global.vi" "LDA Raw Data"() -> (w397:cluster{dbl[][]}[])
            n159 = for {
              tunnel: w397 -> [w416] mode=indexing
              shift-right: [w412] -> w394
              shift-left: w395 -> [w415]
              tunnel: w391 -> [w407]
              shift-right: [w405] -> w393
              shift-left: w390 -> [w406]
              tunnel: w396 -> [w404] mode=indexing
              i -> [w398]
              n160 = Unbundle(w416) -> (w414:dbl[][])
              n161 = Unbundle By Name(w404) -> ("Optics Conversion Factor"=w402:dbl, "Multiply Velocity by -1"=w403:bool)
              n162 = Index Array(array=w414, index (row)=2) -> (element=w400:dbl[])  [unwired: 1 in]
              n163 = Index Array(array=w414, index (row)=0) -> (element=w413:dbl[])  [unwired: 1 in]
              n164 = Index Array(array=w414, index (row)=1) -> (element=w411:dbl[])  [unwired: 1 in]
              n165 = case shown="True" w403 {
                tunnel: w402 -> [w417 w419]
                tunnel: [w417 w418] -> w401
                frame False {
                }
                frame True {
                  n166 = Negate(x=w419) -> (-x=w418:dbl)
                }
              }
              n167 = Multiply(x=w400, y=w401) -> (x*y=w399:dbl[])
              n168 = in-place {
                in-place-border: w413 -> [w433]
                in-place-border: w411 -> [w431]
                in-place-border: w407 -> [w428]
                in-place-border: w399 -> [w424]
                in-place-border: w398 -> [w421]
                n169 = in-place-array #11(w415, w398) -> (w435:T10)
                n170 = in-place-array #12(w406, w398) -> (w423:T8)
                n171 = Unbundle By Name(w423) -> ("Sync Delay Time (s)"=w426:dbl)
                n172 = Equal To 0?(x=w426) -> (x = 0?=w434:bool)
                n173 = case shown="False" w434 {
                  tunnel: [w437 w439] -> w420
                  tunnel: w433 -> [w438 w439]
                  tunnel: w426 -> [w436 _]
                  frame False {
                    n174 = Subtract(x=w438, y=w436) -> (x-y=w437:dbl[])
                  }
                  frame True {
                  }
                }
                n175 = Multiply(x=1000000.0, y=w431) -> (x*y=w430:dbl[])
                n176 = Bundle By Name(cluster=w435, "Weighting"=w430, "Eng Values"=w424) -> (w429:T10)
                n177 = call "Remove_LDA_Spikes.vi"("Current Block Number"=w428, "Analaysis info Cluster"=w423, "Time (s) In"=w420, "Time Trace In"=w429) -> ("Time (s) Out"=w422:dbl[], "Analaysis info Cluster Out"=w425:T8, "Time trace Out"=w427:T10)
                n178 = call "Update Time Trace.vi"("Channel Index"=w421, "Time (s)"=w422) -> ()  [unwired: 1 in]
                n179 = in-place-array #11(w427) -> (w412:T10[])  [unwired: 1 out]
                n180 = in-place-array #12(w425) -> (w405:T8[])  [unwired: 1 out]
              }
            }
          }
        }
        n181 = Select(t="LDA Sync Channel", s=w365, f="LDA_Angular_Alignment_Tweak") -> (s? t:f=w363:string)
      }
      frame "LDA Sync Channel" {
        n182 = for {
          tunnel: w442 -> [w448] mode=indexing
          tunnel: w441 -> [w458]
          tunnel: w442 -> [w455]
          i -> [w457]
          w449 = "Sync"
          n183 = Unbundle By Name(w448) -> ("Req Sample Rate Hz"=w463:dbl, "Inst type"=w461:T1, "Label"=w451:string, "Calib File"=w447:path)
          n184 = Path To String(path=w447) -> (string=w446:string)
          n185 = call "Get_array_values_fr_String.vi"("String Value"=w446) -> ("Numeric Array"=w454:dbl[])  [unwired: 1 out]
          n186 = To Long Integer(number=w454) -> (32bit integer=w453:i32[])
          n187 = String Length(string=w449) -> (length=w452:i32)
          n188 = String Subset(string=w451, length (rest)=w452) -> (substring=w450:string)  [unwired: 1 in]
          n189 = Equal?(x=Inst_type."Raw voltage" ("Inst type"), y=w461) -> (x = y?=w459:bool)
          n190 = Equal?(x=w450, y=w449) -> (x = y?=w460:bool)
          n191 = And(x=w459, y=w460) -> (x .and. y?=w456:bool)
          n192 = case shown="True" w456 {
            tunnel: w463 -> [_ w464]
            tunnel: w458 -> [_ w475]
            tunnel: w457 -> [_ w474]
            tunnel: w453 -> [_ w472]
            tunnel: w455 -> [_ w470]
            tunnel: w448 -> [_ w466]
            frame False {
            }
            frame True {
              n193 = Empty Array?(array=w472) -> (empty?=w473:bool)
              n194 = global read "LDA_global.vi" "Non-coincident"() -> (w479:bool)
              n195 = case shown="False" w473 {
                tunnel: [w482 w484] -> w471
                tunnel: w470 -> [_ w483]
                tunnel: w472 -> [w482 _]
                frame False {
                }
                frame True {
                  n196 = for {
                    tunnel: [w486] -> w484 mode=indexing if=w485
                    tunnel: w483 -> [w487] mode=indexing
                    i -> [w486]
                    n197 = Unbundle By Name(w487) -> ("Inst Array"=w489:T2)
                    n198 = Equal?(x=Instrument_Array."LDA" ("Inst Array"), y=w489) -> (x = y?=w485:bool)
                  }
                }
              }
              n199 = case shown="True" w479 {
                tunnel: [w493 w494] -> w480
                tunnel: w471 -> [_ w501]
                tunnel: w470 -> [_ w499]
                tunnel: [0.0 ("Sync Delay Time (s)") w497] -> w468
                tunnel: w466 -> [w491 _]
                tunnel: [w490 w496] -> w465
                tunnel: w464 -> [_ w496]
                frame False {
                  n200 = global read "LDA_meas_global_1.vi" "Arrival times"() -> (w493:dbl[])
                  n201 = Unbundle By Name(w491) -> ("Av Sampling Rate"=w490:dbl)
                }
                frame True {
                  n202 = Index Array(array=w501, index=0) -> (element=w495:i32)
                  n203 = Index Array(array=w499, index=w495) -> (element=w498:T8)
                  n204 = Unbundle By Name(w498) -> ("Sync Delay Time (s)"=w497:dbl)
                  n205 = call "Get Time Trace.vi"("Channel Index"=w495) -> ("Time (s)"=w494:dbl[])  [unwired: 1 out]
                }
              }
              n206 = Index Array(array=w475, index=w474) -> (element=w478:T10)
              n207 = Unbundle By Name(w478) -> ("Eng Values"=w477:dbl[])
              n208 = call-poly <vilib>:"Mean.vi"("X"=w477) -> ("mean"=w476:dbl)  [unwired: 1 out]
              n209 = Reciprocal(x=w465) -> (1/x=w481:dbl)
              n210 = call "LDA_analogue_start_time_sync_PN.vi"("Pulse high threshold (V)"=w476, "Analogue dt (s)"=w481, "Analogue LDA burst pulse array (s)"=w477, "LDA arrival times (s)"=w480) -> ("LDA start time rel. to Analogue (s)"=w469:dbl)  [unwired: 6 in, 1 out]
              n211 = Add(x=w469, y=w468) -> (x+y=w467:dbl)
              n212 = for {
                tunnel: w467 -> [w505]
                tunnel: w471 -> [w504] mode=indexing
                n213 = call "Get Time Trace.vi"("Channel Index"=w504) -> ("Time (s)"=w503:dbl[])  [unwired: 1 out]
                n214 = Add(x=w505, y=w503) -> (x+y=w502:dbl[])
                n215 = call "Update Time Trace.vi"("Channel Index"=w504, "Time (s)"=w502) -> ()  [unwired: 1 in]
              }
            }
          }
        }
      }
      frame "LDA_Angular_Alignment_Tweak" {
        # "Deg"
        n216 = feedback #13() -> (w518:dbl[])  [unwired: 1 in]
        n217 = case shown="\"1\"" w514 {
          tunnel: [w534 w543 w548 0.0] -> w520
          tunnel: w518 -> [_ w544 w549 w551]
          tunnel: [1 2 3 0] -> w517
          tunnel: [w531 w541 w546 w551] -> w515
          frame "1" {
            n218 = global read "Meas_global.vi" "Pre Setup String"() -> (w529:string)
            n219 = global read "LDA_global.vi" "Number of LDA Chs"() -> (w537:i32)
            n220 = call "Get_Characters_from_string.vi"("Input string"=w529, "Variable name"="LDA_Angular_Alignment_Tweak_Deg") -> ("Status"=w528:enum16{"Char in string", "Char not in string"}, "Value"=w525:string)  [unwired: 1 in]
            n221 = case shown="\"Char not in string\"" w528 {
              tunnel: [w539 w540] -> w527
              tunnel: w525 -> [w538 _]
              tunnel: dbl[] [0.0] ("Numeric Array") -> [_ w540]
              frame "Char in string" {
                n222 = call "Get_array_values_fr_String.vi"("String Value"=w538) -> ("Numeric Array"=w539:dbl[])  [unwired: 1 out]
              }
              frame "Char not in string" {
              }
            }
            n223 = Decrement(x=w537) -> (x-1=w526:i32)
            n224 = Array Subset(array=w527, length=w526) -> (w533:dbl[])  [unwired: 1 in]
            n225 = Array Subset(array=w533, index=1) -> (w531:dbl[])  [unwired: 1 in]
            n226 = Index Array(array=w533) -> (element=w534:dbl)  [unwired: 1 in]
          }
          frame "2" {
            n227 = Array Subset(array=w544, index=1) -> (w541:dbl[])  [unwired: 1 in]
            n228 = Index Array(array=w544) -> (element=w543:dbl)  [unwired: 1 in]
          }
          frame "3" {
            n229 = Array Subset(array=w549, index=1) -> (w546:dbl[])  [unwired: 1 in]
            n230 = Index Array(array=w549) -> (element=w548:dbl)  [unwired: 1 in]
          }
          frame "No match", Default {
          }
        }
        n231 = feedback-in #13(w515) -> ()
        n232 = Not Equal To 0?(x=w520) -> (x != 0?=w519:bool)
        n233 = case shown="True" w519 {
          tunnel: w520 -> [_ w556]
          tunnel: w523 -> [w554 w571]
          tunnel: [w554 w570] -> w522
          tunnel: w517 -> [_ w563]
          tunnel: w506 -> [_ w564]
          frame False {
          }
          frame True {
            n234 = Divide(x=w556, y=180.0 ("value")) -> (x/y=w573:dbl)
            n235 = call "Get Time Trace.vi"("Channel Index"=w563) -> ("Time (s)"=w568:dbl[])  [unwired: 1 out]
            n236 = Multiply(x=w573, y=3.141592653589793) -> (x*y=w572:dbl)
            n237 = Index Array(array=w571) -> (element #1=w577:T10)  [unwired: 2 in, 1 out]
            n238 = Unbundle By Name(w577) -> ("Eng Values"=w576:dbl[])
            n239 = global read "Dynamic_call_global.ph.vi" "Plug in values"() -> (w558:string[])
            n240 = call "Number_2_string.vi"("number"=w556) -> ("String"=w555:string)  [unwired: 1 in]
            n241 = call "Get Time Trace.vi"("Channel Index"=0) -> ("Time (s)"=w567:dbl[])  [unwired: 1 out]
            n242 = in-place {
              in-place-border: w567 -> [w581]
              in-place-border: w576 -> [w580]
              in-place-border: w568 -> [w579]
              in-place-border: w572 -> [w578]
              n243 = in-place-array #14(w571, w563) -> (w583:T10)
              n244 = in-place {
                in-place-border: w581 -> [w592]
                in-place-border: w580 -> [w591]
                in-place-border: w578 -> [w590]
                in-place-border: w579 -> [w587]
                n245 = in-place-cluster #15(w583) -> ("Eng Values"=w589:dbl[])
                n246 = Cosine(x=w590) -> (cos(x)=w586:dbl)
                n247 = Sine(x=w590) -> (sin(x)=w585:dbl)
                n248 = for {
                  tunnel: w592 -> [w604]
                  tunnel: w587 -> [w603] mode=indexing
                  tunnel: w591 -> [w602]
                  tunnel: w589 -> [w601] mode=indexing
                  tunnel: [w597] -> w588 mode=indexing
                  tunnel: w586 -> [w596]
                  tunnel: w585 -> [w595]
                  shift-right: [w593] -> _
                  shift-left: 0.0 -> [w594]
                  n249 = Threshold 1D Array(1:w594, 2:w603, 3:w604) -> (0:w593:dbl)
                  n250 = Interpolate 1D Array(1:w593, 2:w602) -> (0:w600:dbl)
                  n251 = Multiply(x=w601, y=w596) -> (x*y=w598:dbl)
                  n252 = Multiply(x=w600, y=w595) -> (x*y=w599:dbl)
                  n253 = Subtract(x=w598, y=w599) -> (x-y=w597:dbl)
                }
                n254 = in-place-cluster #15("Eng Values"=w588) -> (w582:T10)
              }
              n255 = in-place-array #14(w582) -> (w570:T10[])  [unwired: 1 out]
            }
            n256 = Build Array (concatenate)(w558, w555) -> (w557:string[])
            n257 = Index Array(array=w564, index=w563) -> (element=w562:T8)
            n258 = global write "Dynamic_call_global.ph.vi" "Plug in values"(w557) -> ()
            n259 = Unbundle By Name(w562) -> ("Inst name"=w561:string)
            n260 = global read "Dynamic_call_global.ph.vi" "Plug in titles"() -> (w566:string[])
            n261 = Concatenate Strings(w561, ":Alignment_Tweak:Deg") -> (w559:string)
            n262 = Build Array (concatenate)(w566, w559) -> (w565:string[])
            n263 = global write "Dynamic_call_global.ph.vi" "Plug in titles"(w565) -> ()
          }
        }
        n264 = Array Size(array=w515) -> (size(s)=w516:i32)
        n265 = Greater Than 0?(x=w516) -> (x > 0?=w510:bool)
        n266 = Decimal String To Number(string=w514) -> (number=w513:i32)  [unwired: 2 in, 1 out]
        n267 = Increment(x=w513) -> (x+1=w512:i32)
        n268 = Number To Decimal String(number=w512) -> (decimal integer string=w511:string)  [unwired: 1 in]
        n269 = Select(t="LDA_Angular_Alignment_Tweak", s=w510, f="Create Averaged Channels") -> (s? t:f=w507:string)
      }
      frame "Create Averaged Channels" {
        n270 = for {
          tunnel: w607 -> [w624] mode=indexing
          tunnel: [w625] -> w608 mode=indexing if=w620
          tunnel: [w623] -> w612 mode=indexing
          tunnel: [w622] -> w611 mode=indexing if=w620
          tunnel: [w621] -> w606 mode=indexing if=w620
          i -> [w625]
          n271 = Unbundle By Name(w624) -> ("Inst name"=w623:string)
          n272 = call "Meas Channels to Average.vi"("Analysis_info_cluster"=w624) -> ("Create Av Channel"=w620:bool, "Desired sampling rate"=w621:dbl, "Av Inst name"=w622:string)  [unwired: 7 in, 1 out]
        }
        n273 = for {
          tunnel: w612 -> [w619]
          tunnel: w611 -> [w618] mode=indexing
          tunnel: [w617] -> w609 mode=indexing
          n274 = Search 1D Array(1D array=w619, element=w618) -> (index of element=w617:i32)  [unwired: 1 in]
        }
        n275 = for {
          shift-right: [w627] -> w605
          shift-left: w610 -> [w631]
          tunnel: w609 -> [w626] mode=indexing
          tunnel: w608 -> [w630] mode=indexing
          tunnel: w606 -> [w629] mode=indexing
          n276 = Reciprocal(x=w629) -> (1/x=w628:dbl)
          n277 = in-place {
            in-place-border: w631 -> [w654]
            in-place-border: w630 -> [w653]
            in-place-border: w628 -> [w636]
            in-place-border: w626 -> [w632]
            n278 = in-place-array #16(w631, w626) -> (w639:T10)
            n279 = call "Get Time Trace.vi"("Channel Index"=w653) -> ("Time (s)"=w648:dbl[])  [unwired: 1 out]
            n280 = Index Array(array=w654, index=w653) -> (element=w652:T10)
            n281 = Unbundle By Name(w652) -> ("Eng Values"=w640:dbl[])
            n282 = Array Size(array=w648) -> (size(s)=w651:i32)
            n283 = Decrement(x=w651) -> (x-1=w650:i32)
            n284 = Index Array(array=w648, index #1=0 ("index"), index #2=w650) -> (element #1=w643:dbl, element #2=w646:dbl)
            n285 = Subtract(x=w646, y=w643) -> (x-y=w645:dbl)
            n286 = Divide(x=w645, y=w636) -> (x/y=w644:dbl)
            n287 = Divide(x=w636, y=2.0) -> (x/y=w634:dbl)
            n288 = for {
              N: w644 -> [_]
              tunnel: w648 -> [w670]
              shift-right: [w667] -> _
              shift-left: 0 -> [w666]
              shift-right: [w664] -> _
              shift-left: w643 -> [w661]
              tunnel: w636 -> [w668]
              tunnel: [w665] -> w642 mode=indexing
              tunnel: [w666] -> w641 mode=indexing
              tunnel: w634 -> [w663]
              tunnel: [w662] -> w633 mode=indexing
              n289 = Add(x=w661, y=w668) -> (x+y=w664:dbl)
              n290 = Threshold 1D Array(1:w666, 2:w664, 3:w670) -> (0:w669:dbl)
              n291 = Add(x=w661, y=w663) -> (x+y=w662:dbl)
              n292 = To Long Integer(number=w669) -> (32bit integer=w667:i32)
              n293 = Subtract(x=w667, y=w666) -> (x-y=w665:i32)
            }
            n294 = for {
              tunnel: w642 -> [w656] mode=indexing
              tunnel: w641 -> [w660] mode=indexing
              tunnel: w640 -> [w659]
              tunnel: [w655] -> w638 mode=indexing
              n295 = Array Subset(array=w659, index=w660, length=w656) -> (w658:dbl[])
              n296 = Add Array Elements(numeric array=w658) -> (sum=w657:dbl)
              n297 = Divide(x=w657, y=w656) -> (x/y=w655:dbl)
            }
            n298 = Bundle By Name(cluster=w639, "Eng Values"=w638) -> (w637:T10)
            n299 = call "Update Time Trace.vi"("Channel Index"=w632, "Time (s)"=w633) -> ()  [unwired: 1 in]
            n300 = in-place-array #16(w637) -> (w627:T10[])  [unwired: 1 out]
          }
        }
      }
      frame "Any Pre Analysis Plugins?" {
        n301 = global read "Dynamic_call_global.ph.vi" "Pre_Analysis Plug Ins"() -> (w678:string[])
        n302 = Empty Array?(array=w678) -> (empty?=w677:bool)
        n303 = case shown="False" w677 {
          tunnel: ["Write to Globals" "Add PWA Data"] -> w672
          tunnel: ["Pre_Analysis Plugins" ""] -> w671
          frame False {
          }
          frame True {
          }
        }
      }
      frame "Pre_Analysis Plugins" {
        n304 = global read "Dynamic_call_global.ph.vi" "Pre_Analysis Plug Ins"() -> (w686:string[])
        n305 = for {
          tunnel: w686 -> [w696] mode=indexing
          tunnel: [w696] -> w685 mode=indexing if=w693
          tunnel: [w696] -> w684 mode=indexing if=w695
          n306 = Match Pattern(string=w696, regular expression="7HP") -> (offset past match=w694:i32)  [unwired: 1 in, 3 out]
          n307 = Less Than 0?(x=w694) -> (x < 0?=w693:bool)
          n308 = Not(x=w693) -> (.not. x?=w695:bool)
        }
        n309 = Build Array (concatenate)(w685, w684) -> (w683:string[])
        n310 = for {
          tunnel: w683 -> [w713] mode=indexing
          w710 = FALSE  # Dialog Box (T)
          n311 = call "Plug_in_Directories.vi"() -> ("Pre_Analysis_Plugins"=w704:path)  [unwired: 2 in, 4 out]
          n312 = Build Path(base path=w704, name or relative path=w713) -> (appended path=w708:path)
          n313 = Open VI Reference(type specifier VI Refnum (for type only)=refnum<vi> refnum ("Plug in"), vi path=w708) -> (vi reference=w701:refnum<vi>, error out=w700:errorcluster)  [unwired: 2 in, 2 out]
          n314 = invoke class="VI Interface Type 0" method="FP.Open"(reference=w701, error in=w700, "Activate"=FALSE ("Activate?"), "State"=T3."Standard") -> (reference out=w699:refnum<vi>, error out=w698:errorcluster)  [unwired: 1 in, 3 out]
          n315 = call-by-ref "?"(reference=w699, error in=w698) -> (reference out=w711:refnum<vi>, error out=w712:errorcluster)  [unwired: 1 in]
          n316 = Concatenate Strings("Running Pre_Analysis Plugin named" ("Error Type"), w713) -> (w705:string)
          n317 = Close Reference(reference=w711, error in (no error)=w712) -> (error out=w709:errorcluster)
          n318 = call "EnFlo_Error_Handler.vi"("error in (no error)"=w709, "Error Type"=w705, "Dialog Box (F)"=w710) -> ()  [unwired: 3 out]
        }
      }
      frame "Add PWA Data" {
        n319 = global read "Meas_global.vi" "PWA Data"() -> (w721:T13)
        n320 = case shown="\"One Ch PWA\"" w721 {
          tunnel: [w728 w740] -> w726
          tunnel: [w728 w739] -> w725
          tunnel: [w727 w734] -> w723
          tunnel: [w727 w733] -> w724
          tunnel: [w727 w731] -> w722
          tunnel: w715 -> [_ w729]
          frame "No PWA Data" {
            w727 = 0 ("y")
            w728 = dbl[][] []
          }
          frame "One Ch PWA" {
            n321 = global read "PWAtasksGLOBAL.vi" "PWA Binary"() -> (w730:i16[][])
            n322 = global read "PWAtasksGLOBAL.vi" "Minimum TOF Index"() -> (w738:i16)
            n323 = global read "PWAtasksGLOBAL.vi" "PWA Lookup Table"() -> (w737:dbl[])
            n324 = Equal?(x=w729, y=1) -> (x = y?=w732:bool)
            n325 = Index Array(array=w730, index (row)=0) -> (element=w743:i16[])  [unwired: 1 in]
            n326 = global read "PWAtasksGLOBAL.vi" "PWA Seconds per clock pulse"() -> (w736:dbl)
            n327 = for {
              tunnel: w743 -> [w762] mode=indexing
              tunnel: [w764] -> w742 mode=indexing
              tunnel: [w763] -> w741 mode=indexing
              tunnel: w738 -> [w761]
              tunnel: w737 -> [w760]
              tunnel: w736 -> [w759]
              shift-right: [w758] -> w734
              shift-left: _ -> [w756]
              shift-right: [w757] -> w733
              shift-left: _ -> [w755]
              tunnel: w732 -> [w752]
              shift-right: [w746] -> w731
              shift-left: _ -> [w748]
              i -> [w754]
              w745 = 0 ("y")
              n328 = Equal To 0?(x=w754) -> (x = 0?=w753:bool)
              n329 = And(x=w752, y=w753) -> (x .and. y?=w749:bool)
              n330 = Select(t=w745, s=w749, f=w748) -> (s? t:f=w747:i32)
              n331 = Select(t=w745, s=w749, f=w756) -> (s? t:f=w751:i32)
              n332 = Select(t=w745, s=w749, f=w755) -> (s? t:f=w750:i32)
              n333 = case shown="0, Default" w762 {
                tunnel: w762 -> [w772 _ _]
                tunnel: [w777 w810 w815] -> w764
                tunnel: [w778 w810 w815] -> w763
                tunnel: w761 -> [w776 _ _]
                tunnel: w760 -> [w774 _ _]
                tunnel: w759 -> [w771 _ _]
                tunnel: w751 -> [w770 w809 w814]
                tunnel: [w769 w808 w813] -> w758
                tunnel: [w767 w807 w812] -> w757
                tunnel: w750 -> [w768 w807 w812]
                tunnel: w747 -> [w766 w806 w811]
                tunnel: [w765 w806 w811] -> w746
                frame 0, Default {
                  n334 = Absolute Value(x=w772) -> (abs(x)=w773:i16)
                  n335 = Greater?(x=w773, y=w776) -> (0:w775:bool)
                  n336 = case shown="True" w775 {
                    tunnel: [w783 w799] -> w778
                    tunnel: [w783 w788] -> w777
                    tunnel: w772 -> [_ w798]
                    tunnel: w774 -> [_ w795]
                    tunnel: w771 -> [_ w793]
                    tunnel: w770 -> [w782 w791]
                    tunnel: [w782 w791] -> w769
                    tunnel: w768 -> [w781 w790]
                    tunnel: [w780 w790] -> w767
                    tunnel: w766 -> [w779 w785]
                    tunnel: [w779 w786] -> w765
                    frame False {
                      w783 = nan
                      n337 = Increment(x=w781) -> (x+1=w780:i32)
                    }
                    frame True {
                      n338 = global read "PWAtasksGLOBAL.vi" "Probe Rotated Thro' 180"() -> (w784:bool)
                      n339 = To Double Precision Float(number=w798) -> (double precision float=w794:dbl)
                      n340 = Add(x=w798, y=i16 4095) -> (x+y=w796:i16)
                      n341 = Multiply(x=w793, y=w794) -> (x*y=w792:dbl)
                      n342 = Index Array(array=w795, index=w796) -> (element=w789:dbl)
                      n343 = Reciprocal(x=w792) -> (1/x=w799:dbl)
                      n344 = case shown="True" w784 {
                        tunnel: w789 -> [w803 w805]
                        tunnel: [w803 w804] -> w788
                        frame False {
                        }
                        frame True {
                          n345 = Negate(x=w805) -> (-x=w804:dbl)
                        }
                      }
                      n346 = Less Than 0?(x=w788) -> (x < 0?=w787:bool)
                      n347 = case shown="True" w787 {
                        tunnel: [w800 w802] -> w786
                        tunnel: w785 -> [w800 w801]
                        frame False {
                        }
                        frame True {
                          n348 = Increment(x=w801) -> (x+1=w802:i32)
                        }
                      }
                    }
                  }
                }
                frame 4095 {
                  w810 = 0.0 ("Eng Values")
                  n349 = Increment(x=w809) -> (x+1=w808:i32)
                }
                frame -4095 {
                  w815 = 0.0 ("Eng Values")
                  n350 = Increment(x=w814) -> (x+1=w813:i32)
                }
              }
            }
            n351 = Build Array(w741) -> (w740:dbl[][])
            n352 = Build Array(w742) -> (w739:dbl[][])
          }
        }
        n353 = global write "PWAtasksGLOBAL.vi" "PWA 1/TOF"(w726) -> ()
        n354 = global write "PWAtasksGLOBAL.vi" "PWA No of Reverse samples"(w722) -> ()
        n355 = global write "PWAtasksGLOBAL.vi" "PWA No of  TOF Below Min"(w724) -> ()
        n356 = global write "PWAtasksGLOBAL.vi" "PWA No of  TOF Timeouts"(w723) -> ()
        n357 = global write "PWAtasksGLOBAL.vi" "PWA Data"(w725) -> ()
      }
      frame "Add Extra Data Channels" {
        n358 = global read "Meas_global.vi" "Create_Derived_Channels_by_Arithmetic"() -> (w825:i32[][])
        n359 = global read "Meas_global.vi" "Duplicate_Channels_by_Arithmetic"() -> (w826:i32[][])
        n360 = Build Array (concatenate)(w826, w825) -> (w824:i32[][])
        n361 = Array Size(array=w824) -> (size(s)=w829:i32[])
        n362 = Index Array(array=w829) -> (element=w828:i32)  [unwired: 1 in]
        n363 = Greater Than 0?(x=w828) -> (x > 0?=w827:bool)
        n364 = case shown="False" w827 {
          tunnel: w824 -> [_ w835]
          tunnel: w822 -> [w830 w834]
          tunnel: [w830 w833] -> w823
          tunnel: w821 -> [_ w832]
          tunnel: enum16{"nearest", "linear"}."linear" ("interp. method") -> [_ w831]
          frame False {
          }
          frame True {
            n365 = for {
              tunnel: w835 -> [w863] mode=indexing
              tunnel: w832 -> [w862]
              shift-right: [w858] -> w833
              shift-left: w834 -> [w847]
              tunnel: w831 -> [w836]
              n366 = Index Array(array=w863) -> (element #1=w839:i32, element #2=w861:i32, element #3=w853:i32)  [unwired: 3 in]
              n367 = Absolute Value(x=w853) -> (abs(x)=w846:i32)
              n368 = Absolute Value(x=w861) -> (abs(x)=w840:i32)
              n369 = Index Array(array=w862, index #1=w840, index #2=w846) -> (element #1=w850:T8, element #2=w849:T8)
              n370 = Index Array(array=w847, index #1=w840, index #2=w846) -> (element #1=w844:T10, element #2=w842:T10)
              n371 = call "Get Coincident Pairs.vi"("interp. method"=w836, "Index2"=w846, "Index1"=w840, "Cluster 2"=w849, "Cluster 1"=w850) -> ("Pairs"=w841:cluster{"Cluster":T14, "Cluster":T14, dbl}, "Need to Update"=w848:bool)  [unwired: 5 in]
              n372 = call "Get Time Trace.vi"("Channel Index"=w840) -> ("Time (s)"=w838:dbl[])  [unwired: 1 out]
              n373 = case shown="True" w848 {
                tunnel: [w866 w874] -> w845
                tunnel: w844 -> [w866 w875]
                tunnel: [w865 w869] -> w843
                tunnel: w842 -> [w865 w870]
                tunnel: w841 -> [_ w871]
                tunnel: w838 -> [w864 w873]
                tunnel: [w864 w872] -> w837
                frame False {
                }
                frame True {
                  n374 = Unbundle(w871) -> ("Cluster"=w868:T14, "Cluster"=w867:T14)  [unwired: 1 out]
                  n375 = call "Select indexed values.vi"("Cluster"=w868, "Values"=w873) -> ("Values Out"=w872:dbl[])  [unwired: 1 in]
                  n376 = call "Index Coincident Pairs.vi"("Interpolation method"=w868, "Time Cluster 1"=w875) -> ("Time Cluster 1 Out"=w874:T10)  [unwired: 1 in]
                  n377 = call "Index Coincident Pairs.vi"("Interpolation method"=w867, "Time Cluster 1"=w870) -> ("Time Cluster 1 Out"=w869:T10)  [unwired: 1 in]
                }
              }
              n378 = Unbundle By Name(w843) -> ("Eng Values"=w855:dbl[])
              n379 = Unbundle By Name(w845) -> ("Eng Values"=w857:dbl[])
              n380 = call "Update Time Trace.vi"("Channel Index"=w839, "Time (s)"=w837) -> ()  [unwired: 1 in]
              n381 = Greater Than 0?(x=w861) -> (x > 0?=w860:bool)
              n382 = Greater Than 0?(x=w853) -> (x > 0?=w852:bool)
              n383 = case shown="False" w852 {
                tunnel: [w876 w878] -> w854
                tunnel: w855 -> [w877 w878]
                frame False {
                  n384 = Negate(x=w877) -> (-x=w876:dbl[])
                }
                frame True {
                }
              }
              n385 = case shown="True" w860 {
                tunnel: [w879 w881] -> w856
                tunnel: w857 -> [w880 w881]
                frame False {
                  n386 = Negate(x=w880) -> (-x=w879:dbl[])
                }
                frame True {
                }
              }
              n387 = Add(x=w856, y=w854) -> (x+y=w851:dbl[])
              n388 = Bundle By Name(cluster=w845, "Eng Values"=w851) -> (w859:T10)
              n389 = Replace Array Subset(array=w847, new element=w859, index=w839) -> (w858:T10[])
            }
          }
        }
      }
      frame "Min Max Limiter" {
        n390 = for {
          tunnel: w885 -> [w900] mode=indexing
          tunnel: [w898] -> w890 mode=indexing
          n391 = Unbundle By Name(w900) -> ("Max value"=w903:dbl, "Min value"=w902:dbl)
          n392 = Not A Number/Path/Refnum?(number/path/refnum=w902) -> (NaN/Path/Refnum?=w899:bool)
          n393 = Not A Number/Path/Refnum?(number/path/refnum=w903) -> (NaN/Path/Refnum?=w901:bool)
          n394 = Compound Arithmetic op=OR(invert w901, invert w899) -> (w898:bool)
        }
        n395 = Or Array Elements(Boolean array=w890) -> (logical OR=w889:bool)
        n396 = case shown="True" w889 {
          tunnel: w888 -> [w891 w894]
          tunnel: w885 -> [_ w893]
          tunnel: [w891 w892] -> w887
          frame False {
          }
          frame True {
            n397 = for {
              tunnel: w894 -> [w897] mode=indexing
              tunnel: w893 -> [w896] mode=indexing
              tunnel: [w895] -> w892 mode=indexing
              n398 = call "Max_Min_Limiter.vi"("Analysis info"=w896, "Time Trace In"=w897) -> ("Time Trace Out"=w895:T10)  [unwired: 1 in]
            }
          }
        }
      }
      frame "Analysis of Time Traces" {
        n399 = feedback #17() -> (w909:T15[])  [unwired: 1 in]
        n400 = call "Cluster_Analysis.vi"("Shift In"=w909, "Time Trace in"=w911, "Analysis Info cluster"=w912) -> ("Shift Out"=w910:T15[], "Autocorrelation"=w907:T16[], "Histogram"=w906:T16[], "Analysis Info Cluster Out"=w905:T8[], "Spectra"=w908:T16[], "Error String"=w904:string)  [unwired: 3 in]
        n401 = feedback-in #17(w910) -> ()
        n402 = global write "Meas_global.vi" "Spectra"(w908) -> ()
        n403 = global write "Meas_global.vi" "Histogram"(w906) -> ()
        n404 = global write "Meas_global.vi" "Autocorrelation"(w907) -> ()
        n405 = Concatenate Strings(w917, w904) -> (w916:string)
      }
      frame "Vel Stats Display" {
        n406 = for {
          tunnel: w923 -> [w952] mode=indexing
          tunnel: [w961] -> w932 mode=indexing
          tunnel: [w957] -> w927 mode=indexing
          n407 = Unbundle By Name(w952) -> ("chState"=w950:T9, "Inst name"=w951:string, "Total Meas Time (s)"=w957:dbl, "U"=w956:dbl, "u^2"=w955:dbl, "Av Sampling Rate"=w954:dbl, "Av No of Samples"=w953:dbl, "% u'/U"=w960:dbl, "Sd Error in Mean"=w958:dbl, "Stats"=w959:enum16{"None", "Basic", "Full"})
          n408 = case shown="\"Mute\"" w950 {
            tunnel: [w963 w986] -> w961
            tunnel: w960 -> [_ w984]
            tunnel: w959 -> [_ w979]
            tunnel: w958 -> [_ w976]
            tunnel: w956 -> [_ w975]
            tunnel: w955 -> [_ w974]
            tunnel: w954 -> [_ w973]
            tunnel: w953 -> [_ w970]
            tunnel: w951 -> [w965 w966]
            frame "Mute" {
              w962 = ""
              n409 = Build Array(w965, "Muted" ("element"), w962, w962, w962, w962, w962, w962) -> (w963:string[])
            }
            frame Default {
              n410 = call "Number_2_string.vi"("precision"="4", "number"=w975) -> ("String"=w980:string)
              n411 = call "Number_2_string.vi"("precision"="4", "number"=w974) -> ("String"=w981:string)
              n412 = call "Number_2_string.vi"("precision"="1", "number"=w973) -> ("String"=w972:string)
              n413 = Number To Decimal String(number=w970) -> (decimal integer string=w969:string)  [unwired: 1 in]
              n414 = Number To Fractional String(number=w984, precision (6)=i16 2) -> (F-format string=w983:string)  [unwired: 2 out]
              n415 = case shown="\"Basic\", \"Full\"" w979 {
                tunnel: [w987 w996] -> w978
                tunnel: [w987 w994] -> w977
                tunnel: w976 -> [_ w991]
                tunnel: w975 -> [_ w990]
                frame "None" {
                  w987 = ""
                }
                frame "Basic", "Full" {
                  n416 = Divide(x=w991, y=w990) -> (x/y=w992:dbl)
                  n417 = Multiply(x=w992, y=100.0) -> (x*y=w989:dbl)
                  n418 = call "Number_2_string.vi"("precision"="5", "number"=w991) -> ("String"=w996:string)
                  n419 = Number To Fractional String(number=w989, precision (6)=i16 2) -> (F-format string=w994:string)  [unwired: 2 out]
                }
              }
              n420 = Build Array(w966, w980, w981, w972, w969, w983, w978, w977) -> (w982:string[])
              n421 = for {
                tunnel: [w1000] -> w986 mode=indexing
                tunnel: w982 -> [w997] mode=indexing
                n422 = Equal?(x="NaN", y=w997) -> (x = y?=w1001:bool)
                n423 = Select(t="", s=w1001, f=w997) -> (s? t:f=w1000:string)
              }
            }
          }
        }
        n424 = Index Array(array=w923, index=0) -> (element=w935:T8)
        n425 = Unbundle By Name(w935) -> ("Label"=w937:string, "Inst type"=w936:T1)
        n426 = case shown="\"Raw voltage\", Default" w936 {
          tunnel: ["U" "P" w1004 "U" "C" ("Symbol") "T" ("Symbol") "T" ("Symbol")] -> w934
          tunnel: w937 -> [_ _ w1004 _ _ _ _]
          frame "Propeller anemometer" {
          }
          frame "Pressure Transducer" {
          }
          frame "Raw voltage", Default {
          }
          frame "Hot wire" {
          }
          frame "Fast FID" {
          }
          frame "Thermocouple" {
          }
          frame "Cold wire" {
          }
        }
        n427 = To Lower Case(string=w934) -> (all lower case string=w942:string)
        n428 = To Upper Case(1:w934) -> (0:w944:string)
        n429 = Format Into String(format string="%% %s'/%s", w942, w944) -> (resulting string=w943:string)  [unwired: 2 in, 1 out]
        n430 = Concatenate Strings(w942, "^2") -> (w940:string)
        n431 = Build Array("Inst name", w944, w940, "Hz" ("element"), "Samples" ("element"), w943, "Sd Er", "% Sd Er") -> (w933:string[])
        n432 = global read "Meas_global.vi" "Processing last block?"() -> (w919:bool)
        n433 = Array Max & Min(array=w927) -> (min value=w928:dbl)  [unwired: 3 out]
        n434 = case shown="False" w919 {
          tunnel: ["Sd Error Low Enough?" "Upload Metadata Ch Values"] -> w920
          frame False {
          }
          frame True {
          }
        }
        n435 = Divide(x=w928, y=60.0) -> (x/y=w929:dbl)
        n436 = Build Array (concatenate)(w933, w932) -> (w931:string[][])
        n437 = global write "Meas_global.vi" "Actual Measurement time (min)"(w929) -> ()
        n438 = global write "Meas_global.vi" "Vel stat display"(w931) -> ()
      }
      frame "Sd Error Low Enough?" {
        # "..and the multirun row has valid skip settings in its Extra Commands fiield, and the skip channel has measured long enough to meet its minimum time..."
        # "If we're in a live multirun..."
        n439 = global read "Meas_global.vi" "Post Process"() -> (w1018:T4)
        n440 = Equal?(x=w1018, y=Post_Process."Take New Data" ("Post Process")) -> (x = y?=w1017:bool)
        n441 = Compound Arithmetic op=AND(w1017, invert "Measurement top level?") -> (w1015:bool)
        n442 = case shown="True" w1015 {
          tunnel: ["" ("Instrument Code Name") w1030] -> w1022
          tunnel: [0.0 ("Sd Error Theshold value") w1029] -> w1021
          tunnel: [FALSE w1028] -> w1020
          frame False {
          }
          frame True {
            n443 = global read "Trav_pos_global.vi" "Current Row"() -> (w1031:T17)
            n444 = global read "Meas_global.vi" "Actual Measurement time (min)"() -> (w1038:dbl)
            n445 = Unbundle By Name(w1031) -> ("Extra Commands"=w1032:string)
            n446 = call "Skip_If Sd_Error_Below.vi"("String to Search"=w1032, "Simulate/Run"=User_Specific_mode."Run VI", "Measurement setup Applied?"=FALSE) -> ("Check for Skip?"=w1036:bool, "Instrument Code Name"=w1030:string, "Sd Error Theshold value"=w1029:dbl, "Minimum Measurement time (Sec)"=w1035:dbl)  [unwired: 2 in, 1 out]
            n447 = Multiply(x=w1038, y=60.0) -> (x*y=w1040:dbl)
            n448 = Greater Or Equal?(x=w1040, y=w1035) -> (x >= y?=w1037:bool)
            n449 = Compound Arithmetic op=AND(w1036, w1037) -> (w1028:bool)
          }
        }
        n450 = case shown="True" w1020 {
          tunnel: w1022 -> [_ w1045]
          tunnel: w1021 -> [_ w1044]
          tunnel: [FALSE w1043] -> w1014
          tunnel: w1012 -> [_ w1042]
          frame False {
          }
          frame True {
            # "...then check the standard error against the skip threshold"
            n451 = for {
              tunnel: w1042 -> [w1049] mode=indexing
              tunnel: [w1048] -> w1046 mode=indexing
              n452 = Unbundle By Name(w1049) -> ("Code name"=w1051:string)
              n453 = Match Pattern(string=w1051, regular expression=":") -> (before substring=w1048:string)  [unwired: 4 out]
            }
            n454 = Search 1D Array(1D array=w1046, element=w1045) -> (index of element=w1047:i32)  [unwired: 1 out]
            n455 = case shown="0, Default" w1047 {
              tunnel: w1047 -> [w1057 _]
              tunnel: [w1055 FALSE] -> w1043
              tunnel: w1044 -> [w1054 _]
              tunnel: w1042 -> [w1053 _]
              frame 0, Default {
                n456 = Index Array(array=w1053, index=w1057) -> (element=w1056:T8)
                n457 = Unbundle By Name(w1056) -> ("Sd Error in Mean"=w1052:dbl)
                n458 = Less?(x=w1052, y=w1054) -> (x < y?=w1055:bool)
              }
              frame -1 {
              }
            }
          }
        }
        n459 = case shown="True" w1014 {
          frame False {
          }
          frame True {
            # "Error is small enough so call this the last block"
            n460 = global write "Meas_global.vi" "Processing last block?"(TRUE ("Processing last block?")) -> ()
          }
        }
      }
      frame "Upload Metadata Ch Values" {
        n461 = global read "Meas_global.vi" "Post Process"() -> (w1065:T4)
        n462 = case shown="\"Take New Data\"" w1065 {
          tunnel: w1063 -> [w1078 w1154]
          tunnel: [w1077 w1154] -> w1064
          frame "Take New Data" {
            n463 = for {
              tunnel: w1078 -> [w1096] mode=indexing
              tunnel: [w1095] -> w1077 mode=indexing
              shift-right: [w1085] -> w1072
              shift-left: "" -> [w1084]
              n464 = Unbundle By Name(w1096) -> ("Calib Constants"=w1087:dbl[], "Inst name"=w1083:string, "Metadata Ch Names"=w1082:string[], "Metadata Ch Values"=w1090:string[])
              n465 = for {
                tunnel: w1082 -> [w1098] mode=indexing
                tunnel: [w1097] -> w1081 mode=indexing
                n466 = Match Pattern(string=w1098, regular expression=":") -> (after substring=w1097:string)  [unwired: 1 in, 3 out]
              }
              n467 = Search 1D Array(1D array=w1081, element="FFID:Type") -> (index of element=w1094:i32)  [unwired: 1 out]
              n468 = Search 1D Array(1D array=w1081, element="Control:Unit") -> (index of element=w1091:i32)  [unwired: 1 out]
              n469 = Index Array(array=w1090, index=w1094) -> (element=w1093:string)
              n470 = Index Array(array=w1090, index=w1091) -> (element=w1089:string)
              n471 = Equal?(x="HFR500", y=w1093) -> (x = y?=w1088:bool)
              n472 = case shown="True" w1088 {
                tunnel: w1096 -> [w1101 w1128]
                tunnel: [w1101 w1127] -> w1095
                tunnel: w1083 -> [_ w1114]
                tunnel: w1089 -> [_ w1126]
                tunnel: w1087 -> [_ w1120]
                tunnel: "The %s %s was %.1f during Calibration, but now is %.1f deg C.\n\n" ("format string") -> [_ w1115]
                tunnel: [w1100 w1112] -> w1085
                tunnel: w1084 -> [w1100 w1110]
                frame False {
                }
                frame True {
                  n473 = call "HFR500 Black Box Path.vi"("Channel Name String"=w1126) -> ("Black Box Path"=w1125:path)  [unwired: 1 in, 1 out]
                  n474 = call "Get Black Box File Data.vi"("Delete File?"=TRUE, "Inst Name"=w1114, "Black Box Filename"=w1125) -> ("Channel Values"=w1106:string[], "Channel Names"=w1109:string[])
                  n475 = for {
                    tunnel: w1109 -> [w1150] mode=indexing
                    tunnel: [w1149] -> w1124 mode=indexing
                    n476 = Reverse String(1:w1150) -> (0:w1153:string)
                    n477 = Match Pattern(string=w1153, regular expression=":") -> (before substring=w1151:string)  [unwired: 1 in, 3 out]
                    n478 = Reverse String(1:w1151) -> (0:w1149:string)
                  }
                  n479 = Array Subset(array=w1120, index=14, length=2) -> (w1103:dbl[])
                  n480 = Build Array("Head(C)", "Exhaust(C)") -> (w1121:string[])
                  n481 = Build Array("Head Temp", "Exhaust Temp") -> (w1113:string[])
                  n482 = for {
                    tunnel: w1124 -> [w1148]
                    tunnel: w1106 -> [w1146]
                    tunnel: w1121 -> [w1144] mode=indexing
                    tunnel: w1103 -> [w1136] mode=indexing
                    tunnel: [w1134] -> w1111 mode=concatenating if=w1138
                    tunnel: w1115 -> [w1137]
                    tunnel: w1114 -> [w1133]
                    tunnel: w1113 -> [w1132] mode=indexing
                    tunnel: [w1130] -> w1108 mode=indexing
                    n483 = Search 1D Array(1D array=w1148, element=w1144) -> (index of element=w1147:i32)  [unwired: 1 in]
                    n484 = Not Equal To 0?(x=w1136) -> (x != 0?=w1139:bool)
                    n485 = Index Array(array=w1146, index=w1147) -> (element=w1145:string)
                    n486 = Fract/Exp String To Number(string=w1145) -> (number=w1135:dbl)  [unwired: 3 in, 1 out]
                    n487 = Subtract(x=w1135, y=w1136) -> (x-y=w1143:dbl)
                    n488 = Absolute Value(x=w1143) -> (abs(x)=w1142:dbl)
                    n489 = Format Into String(format string=w1137, w1133, w1132, w1136, w1135) -> (resulting string=w1134:string)  [unwired: 2 in, 1 out]
                    n490 = Greater?(x=w1142, y=5.0) -> (0:w1140:bool)
                    n491 = And(x=w1140, y=w1139) -> (x .and. y?=w1138:bool)
                    n492 = Format Into String(format string="%s:Calib:%s", w1133, w1132) -> (resulting string=w1130:string)  [unwired: 2 in, 1 out]
                  }
                  n493 = Build Array (concatenate)(w1109, w1108) -> (w1107:string[])
                  n494 = Number To Fractional String(number=w1103, precision (6)=i16 1) -> (F-format string=w1102:string[])  [unwired: 2 in]
                  n495 = Build Array (concatenate)(w1106, w1102) -> (w1105:string[])
                  n496 = call "Update Metadata channels.vi"("Metadata Values"=w1105, "Metadata Names"=w1107, "Analysis info Cluster in"=w1128) -> ("Analysis info Cluster out"=w1127:T8)
                  n497 = Concatenate Strings(w1110, w1111) -> (w1112:string)
                }
              }
            }
            n498 = Empty String/Path?(string/path=w1072) -> (empty?=w1074:bool)
            n499 = Not(x=w1074) -> (.not. x?=w1073:bool)
            n500 = Bundle By Name(cluster=errorcluster {"status"=FALSE, "code"=0, "source"=""} ("error in (no error)"), "source"=w1072, "status"=w1073) -> (w1071:errorcluster)
            n501 = call "EnFlo_Error_Handler.vi"("error in (no error)"=w1071, "Error Type"="FFID Temp", "Dialog Box (F)"=FALSE) -> ()  [unwired: 1 in, 2 out]
          }
          frame "Post Process Raw Data File" {
          }
        }
        n502 = global read "Meas_global.vi" "Over/Under string"() -> (w1061:string)
        n503 = Concatenate Strings(w1061, w1068) -> (w1062:string)
        n504 = global write "Meas_global.vi" "Over/Under string"(w1062) -> ()
      }
      frame "Per Block Plug ins" {
        n505 = global read "Meas_global.vi" "Repeat Measurement?"() -> (w1157:bool)
        n506 = Array Size(array=w1159) -> (size(s)=w1166:i32)
        n507 = Greater Than 0?(x=w1166) -> (x > 0?=w1158:bool)
        n508 = Compound Arithmetic op=AND(w1158, invert w1157) -> (w1156:bool)
        n509 = case shown="True" w1156 {
          tunnel: w1159 -> [_ w1170]
          tunnel: [w1167 "Read from Globals"] -> w1162
          tunnel: ["" w1169] -> w1161
          tunnel: "Voltage Overflows" -> [w1167 w1169]
          frame False {
          }
          frame True {
            n510 = call "Call_Block_plug_ins.vi"("Per Block Plug Ins"=w1170) -> ()
          }
        }
      }
      frame "Voltage Overflows" {
        n511 = stacked-sequence {
          seq-local: [w1186 _ _] -> [_ w1259 _]
          seq-local: [w1185 _ _] -> [_ w1258 _]
          tunnel: [_ _ w1332] -> w1181
          tunnel: w1180 -> [_ _ w1332]
          tunnel: w1179 -> [w1184 w1257 w1330]
          tunnel: [_ _ w1330] -> w1178
          tunnel: [_ _ w1331] -> w1177
          tunnel: w1176 -> [w1183 _ w1331]
          tunnel: w1175 -> [w1182 w1256 _]
          tunnel: [_ "Cross Moments" _] -> w1174
          tunnel: [_ TRUE _] -> w1173
          tunnel: [_ "" _] -> w1172
          frame #0 {
            n512 = Array Size(array=w1184) -> (size(s)=w1191:i32)
            n513 = feedback #18() -> (w1189:i32[])  [unwired: 1 in]
            n514 = feedback #19() -> (w1190:i32[])  [unwired: 1 in]
            n515 = case shown="1" w1182 {
              tunnel: w1191 -> [_ w1196]
              tunnel: [w1193 w1194] -> w1188
              tunnel: w1189 -> [w1193 _]
              tunnel: [w1192 w1194] -> w1187
              tunnel: w1190 -> [w1192 _]
              frame Default {
              }
              frame 1 {
                n516 = Initialize Array(0 ("element"), w1196) -> (w1194:i32[])
              }
            }
            n517 = for {
              tunnel: w1183 -> [w1205] mode=indexing
              tunnel: [w1203] -> w1186 mode=indexing
              tunnel: [w1201] -> w1185 mode=indexing
              tunnel: w1188 -> [w1200] mode=indexing
              tunnel: w1187 -> [w1199] mode=indexing
              tunnel: w1184 -> [w1197] mode=indexing
              n518 = Unbundle By Name(w1197) -> ("Device"=w1198:string)
              n519 = case shown="\"Na-DAS_7609.vi\"" w1198 {
                tunnel: [FALSE TRUE TRUE TRUE TRUE TRUE] -> w1208
                tunnel: [0.0 ("Min") -10.6 ("Min") -9.99 ("Min") -9.99 ("Min") -9.99 ("Min") -9.99 ("Min")] -> w1207
                tunnel: [0.0 ("Max") 10.6 ("Max") 9.99 ("Max") 9.99 ("Max") 9.99 ("Max") 9.99 ("Max")] -> w1206
                frame Default {
                }
                frame "Na-DAS_7609.vi" {
                }
                frame "NI-DAQmx.vi" {
                }
                frame "NI-DAQmxBaseKernel.vi" {
                }
                frame "DataTranslation.vi" {
                }
                frame "DT_With_Multiplexer.vi" {
                }
              }
              n520 = case shown="True" w1208 {
                tunnel: [0 w1217] -> w1204
                tunnel: [0 w1215] -> w1202
                tunnel: w1207 -> [_ w1214]
                tunnel: w1206 -> [_ w1213]
                tunnel: w1205 -> [_ w1212]
                frame False {
                }
                frame True {
                  n521 = Unbundle By Name(w1212) -> ("Voltage"=w1211:dbl[])
                  n522 = Array Max & Min(array=w1211) -> (max value=w1220:dbl, min value=w1219:dbl)  [unwired: 2 out]
                  n523 = Less?(x=w1220, y=w1213) -> (x < y?=w1218:bool)
                  n524 = Greater?(x=w1219, y=w1214) -> (0:w1216:bool)
                  n525 = case shown="False" w1218 {
                    tunnel: w1211 -> [w1233 _]
                    tunnel: w1213 -> [w1232 _]
                    tunnel: [w1229 0] -> w1217
                    frame False {
                      n526 = Greater?(x=w1233, y=w1232) -> (0:w1231:bool[])
                      n527 = Boolean To (0,1)(Boolean=w1231) -> (0, 1=w1230:i16[])
                      n528 = To Long Integer(number=w1230) -> (32bit integer=w1228:i32[])
                      n529 = Add Array Elements(numeric array=w1228) -> (sum=w1229:i32)
                    }
                    frame True {
                    }
                  }
                  n530 = case shown="False" w1216 {
                    tunnel: w1211 -> [w1226 _]
                    tunnel: w1214 -> [w1225 _]
                    tunnel: [w1222 0] -> w1215
                    frame False {
                      n531 = Less?(x=w1226, y=w1225) -> (x < y?=w1224:bool[])
                      n532 = Boolean To (0,1)(Boolean=w1224) -> (0, 1=w1223:i16[])
                      n533 = To Long Integer(number=w1223) -> (32bit integer=w1221:i32[])
                      n534 = Add Array Elements(numeric array=w1221) -> (sum=w1222:i32)
                    }
                    frame True {
                    }
                  }
                }
              }
              n535 = Add(x=w1204, y=w1200) -> (x+y=w1203:i32)
              n536 = Add(x=w1202, y=w1199) -> (x+y=w1201:i32)
            }
            n537 = feedback-in #18(w1186) -> ()
            n538 = feedback-in #19(w1185) -> ()
          }
          frame #1 {
            n539 = Add Array Elements(numeric array=w1258) -> (sum=w1266:i32)
            n540 = Add Array Elements(numeric array=w1259) -> (sum=w1265:i32)
            n541 = Greater Than 0?(x=w1266) -> (x > 0?=w1264:bool)
            n542 = Greater Than 0?(x=w1265) -> (x > 0?=w1263:bool)
            n543 = global read "Meas_global.vi" "Processing last block?"() -> (w1261:bool)
            n544 = Or(x=w1263, y=w1264) -> (x .or. y?=w1262:bool)
            n545 = And(x=w1261, y=w1262) -> (x .and. y?=w1260:bool)
            n546 = case shown="True" w1260 {
              tunnel: w1259 -> [_ w1276]
              tunnel: w1256 -> [_ w1275]
              tunnel: w1258 -> [_ w1274]
              tunnel: w1257 -> [_ w1269]
              frame False {
              }
              frame True {
                n547 = global read "Meas_global.vi" "Over/Under string"() -> (w1273:string)
                n548 = global read "Meas_global.vi" "Extra Comments"() -> (w1270:string)
                n549 = global read "Meas_global.vi" "Iteration Number"() -> (w1268:i32)
                n550 = Equal To 0?(x=w1268) -> (x = 0?=w1267:bool)
                n551 = for {
                  tunnel: w1276 -> [w1296] mode=indexing
                  tunnel: w1269 -> [w1310] mode=indexing
                  tunnel: w1275 -> [w1308]
                  tunnel: w1274 -> [w1297] mode=indexing
                  shift-right: [w1292] -> w1272
                  shift-left: w1273 -> [w1293]
                  shift-right: [w1294] -> w1271
                  shift-left: w1270 -> [w1295]
                  tunnel: w1267 -> [w1281]
                  n552 = Unbundle By Name(w1310) -> ("Inst name"=w1299:string, "Av No of Samples"=w1309:dbl, "Device"=w1282:string)
                  n553 = Greater Than 0?(x=w1297) -> (x > 0?=w1279:bool)
                  n554 = Greater Than 0?(x=w1296) -> (x > 0?=w1278:bool)
                  n555 = Multiply(x=w1309, y=w1308) -> (x*y=w1303:dbl)
                  n556 = Divide(x=w1296, y=w1303) -> (x/y=w1307:dbl)
                  n557 = Divide(x=w1297, y=w1303) -> (x/y=w1304:dbl)
                  n558 = Multiply(x=w1304, y=100.0) -> (x*y=w1298:dbl)
                  n559 = Multiply(x=w1307, y=100.0) -> (x*y=w1301:dbl)
                  n560 = Equal?(x=w1282, y="Na-DAS_7609.vi") -> (x = y?=w1280:bool)
                  n561 = Greater?(x=w1301, y=0.02) -> (0:w1291:bool)
                  n562 = case shown="True" w1278 {
                    tunnel: w1301 -> [_ w1328]
                    tunnel: w1299 -> [_ w1327]
                    tunnel: ["" w1326] -> w1289
                    frame False {
                    }
                    frame True {
                      n563 = Format Into String(format string="%s has %.3f%% Overflows at ADC.\\n" ("Format String"), w1327, w1328) -> (resulting string=w1326:string)  [unwired: 2 in, 1 out]
                    }
                  }
                  n564 = Compound Arithmetic op=AND(w1278, w1279, w1280, w1281) -> (w1277:bool)
                  n565 = case shown="True" w1279 {
                    tunnel: w1298 -> [_ w1321]
                    tunnel: w1299 -> [_ w1323]
                    tunnel: ["" w1322] -> w1287
                    frame False {
                    }
                    frame True {
                      n566 = Format Into String(format string="%s has %.3f%% Underflows at ADC.\n" ("Format String"), w1323, w1321) -> (resulting string=w1322:string)  [unwired: 2 in, 1 out]
                    }
                  }
                  n567 = Greater?(x=w1298, y=0.02) -> (0:w1286:bool)
                  n568 = case shown="False" w1277 {
                    frame False {
                    }
                    frame True {
                      n569 = global write "Meas_global.vi" "Repeat Measurement?"(TRUE ("Repeat Measurement?")) -> ()
                    }
                  }
                  n570 = case shown="True" w1291 {
                    tunnel: ["" w1319] -> w1290
                    tunnel: w1289 -> [w1316 w1319]
                    tunnel: [w1316 ""] -> w1288
                    frame False {
                    }
                    frame True {
                    }
                  }
                  n571 = case shown="False" w1286 {
                    tunnel: ["" w1315] -> w1285
                    tunnel: w1287 -> [w1312 w1315]
                    tunnel: [w1312 ""] -> w1284
                    frame False {
                    }
                    frame True {
                    }
                  }
                  n572 = Concatenate Strings(w1295, w1288, w1284) -> (w1294:string)
                  n573 = Concatenate Strings(w1293, w1290, w1285) -> (w1292:string)
                }
                "Extra Comments" <- w1271
                "Over/Under string" <- w1272
                n574 = global write "Meas_global.vi" "Over/Under string"(w1272) -> ()
                n575 = global write "Meas_global.vi" "Extra Comments"(w1271) -> ()
              }
            }
          }
          frame #2 {
          }
        }
      }
      frame "Cross Moments" {
        n576 = global read "Meas_global.vi" "Duplicate Chs to correlate"() -> (w1351:i32[][])
        n577 = global read "Meas_global.vi" "correlate"() -> (w1352:i32[][])
        n578 = Build Array (concatenate)(w1352, w1351) -> (w1339:i32[][])
        n579 = Array Size(array=w1339) -> (size(s)=w1349:i32[])
        n580 = Index Array(array=w1349) -> (element=w1348:i32)  [unwired: 1 in]
        n581 = call "Split Array index for Parallel Code.vi"("Array Size"=w1348) -> ("Length3"=w1342:i32, "Index3"=w1343:i32, "Length2"=w1344:i32, "Index2"=w1345:i32, "Index4"=w1341:i32, "Length1"=w1346:i32, "Length4"=w1340:i32, "Index1"=w1347:i32)  [unwired: 3 in]
        n582 = Array Subset(array=w1339, index (row)=w1341, length (row)=w1340) -> (w1333:i32[][])  [unwired: 2 in]
        n583 = Array Subset(array=w1339, index (row)=w1345, length (row)=w1344) -> (w1335:i32[][])  [unwired: 2 in]
        n584 = Array Subset(array=w1339, index (row)=w1343, length (row)=w1342) -> (w1334:i32[][])  [unwired: 2 in]
        n585 = Array Subset(array=w1339, index (row)=w1347, length (row)=w1346) -> (w1338:i32[][])  [unwired: 2 in]
        n586 = while {
          shift-right: [w1367] -> _
          shift-left: _ -> [w1368]
          shift-right: [w1365] -> _
          shift-left: _ -> [w1366]
          shift-right: [w1380] -> _
          shift-left: _ -> [w1381]
          shift-right: [w1378] -> _
          shift-left: _ -> [w1379]
          shift-right: [w1363] -> _
          shift-left: _ -> [w1364]
          shift-right: [w1361] -> _
          shift-left: _ -> [w1362]
          shift-right: [w1359] -> _
          shift-left: _ -> [w1360]
          shift-right: [w1357] -> _
          shift-left: _ -> [w1358]
          tunnel: [w1383] -> w1350
          tunnel: w1338 -> [w1382]
          tunnel: w1337 -> [w1373]
          tunnel: w1336 -> [w1372]
          tunnel: w1335 -> [w1376]
          tunnel: w1334 -> [w1375]
          tunnel: w1333 -> [w1374]
          stop <- TRUE stop-if-true
          n587 = call "WeightedCrossMomentsWrapped.vi"("Shift2In"=w1366, "Shift1In"=w1368, "IndicesIn"=w1376, "Time Trace in"=w1372, "Analysis Info clusterIn"=w1373) -> ("Shift1Out"=w1367:T20[], "ResultsOut"=w1371:T21[], "Shift2Out"=w1365:T15[])  [unwired: 4 in]
          n588 = call "WeightedCrossMomentsWrapped.vi"("Shift2In"=w1379, "Shift1In"=w1381, "IndicesIn"=w1382, "Time Trace in"=w1372, "Analysis Info clusterIn"=w1373) -> ("Shift1Out"=w1380:T20[], "ResultsOut"=w1377:T21[], "Shift2Out"=w1378:T15[])  [unwired: 4 in]
          n589 = call "WeightedCrossMomentsWrapped.vi"("Shift2In"=w1362, "Shift1In"=w1364, "IndicesIn"=w1375, "Time Trace in"=w1372, "Analysis Info clusterIn"=w1373) -> ("Shift1Out"=w1363:T20[], "ResultsOut"=w1370:T21[], "Shift2Out"=w1361:T15[])  [unwired: 4 in]
          n590 = call "WeightedCrossMomentsWrapped.vi"("Shift2In"=w1358, "Shift1In"=w1360, "IndicesIn"=w1374, "Time Trace in"=w1372, "Analysis Info clusterIn"=w1373) -> ("Shift1Out"=w1359:T20[], "ResultsOut"=w1369:T21[], "Shift2Out"=w1357:T15[])  [unwired: 4 in]
          n591 = Build Array (concatenate)(w1377, w1371, w1370, w1369) -> (w1383:T21[])
        }
        n592 = global write "Meas_global.vi" "Correlation Results"(w1350) -> ()
      }
      frame "Output Cross moments" {
        n593 = global read "Meas_global.vi" "Correlation Results"() -> (w1395:T21[])
        n594 = global read "Meas_global.vi" "Vel stat display"() -> (w1392:string[][])
        n595 = Array Size(array=w1395) -> (size(s)=w1394:i32)
        n596 = Greater Than 0?(x=w1394) -> (x > 0?=w1393:bool)
        n597 = case shown="True" w1393 {
          tunnel: w1395 -> [_ w1405]
          tunnel: w1392 -> [w1396 w1398]
          tunnel: [w1396 w1397] -> w1391
          frame False {
          }
          frame True {
            n598 = for {
              tunnel: [w1412] -> w1400 mode=indexing
              tunnel: w1405 -> [w1411] mode=indexing
              n599 = Unbundle By Name(w1411) -> ("U inst"=w1414:string, "W inst"=w1413:string, "uw"=w1407:dbl, "uw/u'w'"=w1409:dbl)
              n600 = call "Number_2_string.vi"("number"=w1407) -> ("String"=w1406:string)  [unwired: 1 in]
              n601 = Number To Fractional String(number=w1409, precision (6)=i16 3) -> (F-format string=w1408:string)  [unwired: 2 out]
              n602 = Build Array(w1414, w1413, w1406, w1408) -> (w1412:string[])
            }
            n603 = Build Array("u inst", "w inst", "uw", "uw/u'w'") -> (w1399:string[])
            n604 = Build Array (concatenate)(w1398, w1399, w1400) -> (w1397:string[][])
          }
        }
        "Vel stat display" <- w1391
        n605 = global write "Meas_global.vi" "Vel stat display"(w1391) -> ()
      }
      frame "Create Plot Clusters" {
        n606 = global read "Meas_global.vi" "Second Graph"() -> (w1417:T23)
        n607 = global read "Meas_global.vi" "First Graph"() -> (w1416:T23)
        n608 = global read "Meas_global.vi" "File"() -> (w1422:T6)
        n609 = Not Equal?(x=T6."Save no data" ("File"), y=w1422) -> (x != y?=w1423:bool)
        n610 = Build Array(w1416, w1417) -> (w1415:T24)
        n611 = for {
          tunnel: w1423 -> [w1448]
          tunnel: w1420 -> [w1438]
          tunnel: "No of estimates output" -> [w1437]
          tunnel: w1418 -> [w1436]
          tunnel: w1415 -> [w1433] mode=indexing
          i -> [w1435]
          n612 = Unbundle By Name(w1433) -> ("Plot 1"=w1445:u16, "Plot 2"=w1444:u16, "Plot Type"=w1440:T22, "Save graph"=w1443:u16)
          n613 = case shown="\"Show no graph\"" w1440 {
            tunnel: [FALSE TRUE TRUE w1457] -> w1439
            frame "Show no graph" {
            }
            frame "Voltage trace" {
            }
            frame "Velocity trace" {
            }
            frame "Vel histogram", Default {
              n614 = global read "Meas_global.vi" "Processing last block?"() -> (w1457:bool)
            }
          }
          n615 = Build Array(w1445, w1444) -> (w1431:u16[])
          n616 = for {
            tunnel: w1431 -> [w1451] mode=indexing
            tunnel: [w1450] -> w1430 mode=indexing if=w1449
            n617 = Not Equal To 0?(x=w1451) -> (x != 0?=w1449:bool)
            n618 = Decrement(x=w1451) -> (x-1=w1450:u16)
          }
          n619 = Equal?(x=w1443, y=u16 1 ("Save graph")) -> (x = y?=w1441:bool)
          n620 = global read "Meas_global.vi" "Spectra"() -> (w1432:T16[])
          n621 = And(x=w1441, y=w1439) -> (x .and. y?=w1446:bool)
          n622 = And(x=w1446, y=w1448) -> (x .and. y?=w1447:bool)
          n623 = for {
            tunnel: w1440 -> [w1466]
            tunnel: [w1463] -> w1434 mode=indexing
            tunnel: w1447 -> [w1467]
            tunnel: w1437 -> [w1464]
            tunnel: w1438 -> [w1462]
            tunnel: w1436 -> [w1458]
            tunnel: w1432 -> [w1460]
            tunnel: w1430 -> [w1459] mode=indexing
            n624 = case shown="\"Voltage trace\"" w1466 {
              tunnel: [w1477 w1483 w1491 w1501 w1506 w1512 w1517] -> w1470
              tunnel: [w1477 w1486 w1496 w1500 w1505 w1510 w1516] -> w1469
              tunnel: w1459 -> [_ w1482 w1492 w1499 w1504 w1509 w1514]
              tunnel: w1462 -> [_ w1484 w1494 _ _ _ _]
              tunnel: [_ _ w1493 _ _ _ _] -> w1461
              tunnel: w1460 -> [_ _ _ _ w1502 w1507 _]
              tunnel: w1458 -> [_ w1481 _ _ _ _ _]
              frame "Show no graph" {
                w1477 = dbl[] [] ("X array")
              }
              frame "Voltage trace" {
                n625 = Index Array(array=w1481, index=w1482) -> (element=w1480:T8)
                n626 = Index Array(array=w1484, index=w1482) -> (element=w1485:T10)
                n627 = Unbundle By Name(w1480) -> ("Inst type"=w1479:T1)
                n628 = call "Data Type for Instrument.vi"("Inst type"=w1479) -> ("Data for Inst Type"=w1478:T25)
                n629 = case shown="\"Eng Values\"" w1478 {
                  tunnel: [w1488 w1490] -> w1486
                  tunnel: w1485 -> [w1487 w1489]
                  frame "Voltage" {
                    n630 = Unbundle By Name(w1487) -> ("Voltage"=w1488:dbl[])
                  }
                  frame "Eng Values" {
                    n631 = Unbundle By Name(w1489) -> ("Eng Values"=w1490:dbl[])
                  }
                }
                n632 = call "Get Time Trace.vi"("Channel Index"=w1482) -> ("Time (s)"=w1483:dbl[])  [unwired: 1 out]
              }
              frame "Velocity trace" {
                n633 = Index Array(array=w1494, index=w1492) -> (element=w1495:T10)
                n634 = Unbundle By Name(w1495) -> ("Eng Values"=w1496:dbl[], "Weighting"=w1493:dbl[])
                n635 = call "Get Time Trace.vi"("Channel Index"=w1492) -> ("Time (s)"=w1491:dbl[])  [unwired: 1 out]
              }
              frame "Vel histogram" {
                n636 = global read "Meas_global.vi" "Histogram"() -> (w1497:T16[])
                n637 = Index Array(array=w1497, index=w1499) -> (element=w1498:T16)
                n638 = Unbundle By Name(w1498) -> ("X array"=w1501:dbl[], "Y array"=w1500:dbl[])
              }
              frame "Spectrum" {
                n639 = Index Array(array=w1502, index=w1504) -> (element=w1503:T16)
                n640 = Unbundle By Name(w1503) -> ("X array"=w1506:dbl[], "Y array"=w1505:dbl[])
              }
              frame "f.E(f) v Log f" {
                n641 = Index Array(array=w1507, index=w1509) -> (element=w1508:T16)
                n642 = Unbundle By Name(w1508) -> ("X array"=w1512:dbl[], "Y array"=w1511:dbl[])
                n643 = Multiply(x=w1512, y=w1511) -> (x*y=w1510:dbl[])
              }
              frame "Auto-Corr" {
                n644 = global read "Meas_global.vi" "Autocorrelation"() -> (w1515:T16[])
                n645 = Index Array(array=w1515, index=w1514) -> (element=w1513:T16)
                n646 = Unbundle By Name(w1513) -> ("X array"=w1517:dbl[], "Y array"=w1516:dbl[])
              }
            }
            n647 = Greater Or Equal To 0?(x=w1459) -> (x >= 0?=w1468:bool)
            n648 = And(x=w1468, y=w1467) -> (x .and. y?=w1465:bool)
            n649 = Bundle("X array"=w1470, "Y array"=w1469) -> (w1463:cluster{"X array":dbl[], "Y array":dbl[]})  [unwired: 1 in]
            n650 = case shown="True" w1465 {
              tunnel: w1466 -> [_ w1476]
              tunnel: w1459 -> [_ w1475]
              tunnel: w1464 -> [_ w1474]
              tunnel: w1463 -> [_ w1473]
              tunnel: w1458 -> [_ w1472]
              tunnel: w1461 -> [_ w1471]
              frame False {
              }
              frame True {
                n651 = call "Save_Data.vi"("Analysis Info cluster"=w1472, "Plot Data"=w1473, "No of estimates output"=w1474, "Index"=w1475, "Weighting"=w1471, "Plot Type"=w1476) -> ()  [unwired: 1 in]
              }
            }
          }
          n652 = case shown="0, Default" w1435 {
            tunnel: w1434 -> [w1452 w1453]
            frame 0, Default {
              "First Plot data Cluster" <- w1452
            }
            frame 1 {
              "Second Plot Data Cluster" <- w1453
            }
          }
        }
        n653 = global read "Meas_global.vi" "LDA data"() -> (w1427:enum16{"No LDA data", "Take LDA data"})
        n654 = Equal?(x=w1427, y=enum16{"No LDA data", "Take LDA data"}."Take LDA data" ("LDA data")) -> (x = y?=w1426:bool)
      }
      frame "Seeder Control?" {
        n655 = global read "Preference_global.vi" "Server Comms"() -> (w1525:T7)
        n656 = global read "Meas_global.vi" "Post Process"() -> (w1522:T4)
        n657 = global read "Meas_global.vi" "File"() -> (w1528:T6)
        n658 = Equal?(x=w1528, y=T6."Save no data" ("File")) -> (x = y?=w1530:bool)
        n659 = Equal?(x=w1522, y=Post_Process."Take New Data" ("Post Process")) -> (x = y?=w1527:bool)
        n660 = Equal?(x=w1525, y=Server_Comms."Server Link Healthy" ("Server Comms")) -> (x = y?=w1526:bool)
        n661 = Compound Arithmetic op=AND(invert w1530, w1527, w1526) -> (w1531:bool)
      }
      frame "Control Seeding level" {
        # "Req Sampling Rate"
        # "Av Sampling Rate"
        n662 = stacked-sequence {
          seq-local: [w1546 _] -> [_ w1560]
          seq-local: [w1543 _] -> [_ w1561]
          seq-local: [w1540 _] -> [_ w1559]
          tunnel: w1536 -> [w1539 _]
          frame #0 {
            n663 = for {
              tunnel: w1539 -> [w1558] mode=indexing
              tunnel: [w1555] -> w1542 mode=indexing if=w1548
              tunnel: [w1554] -> w1547 mode=indexing if=w1548
              tunnel: [w1553] -> w1545 mode=indexing if=w1548
              n664 = Unbundle By Name(w1558) -> ("Inst type"=w1557:T1, "Av Sampling Rate"=w1554:dbl, "Req Sample Rate Hz"=w1553:dbl, "Av No of Samples"=w1552:dbl)
              n665 = Greater?(x=w1552, y=5.0) -> (0:w1549:bool)
              n666 = Equal?(x=Inst_type."LDA Vel" ("Inst type"), y=w1557) -> (x = y?=w1550:bool)
              n667 = Divide(x=w1554, y=w1553) -> (x/y=w1555:dbl)
              n668 = And(x=w1550, y=w1549) -> (x .and. y?=w1548:bool)
            }
            n669 = Array Size(array=w1542) -> (size(s)=w1541:i32)
            n670 = Array Max & Min(array=w1542) -> (min index (indices)=w1544:i32)  [unwired: 3 out]
            n671 = Greater Than 0?(x=w1541) -> (x > 0?=w1540:bool)
            n672 = Index Array(array=w1547, index=w1544) -> (element=w1546:dbl)
            n673 = Index Array(array=w1545, index=w1544) -> (element=w1543:dbl)
          }
          frame #1 {
            w1563 = 2.0 ("y")
            n674 = Greater?(x=w1560, y=w1563) -> (0:w1564:bool)
            n675 = global read "Preference_global.vi" "Rig Setup"() -> (w1565:string)
            n676 = Select(t=w1560, s=w1564, f=w1563) -> (s? t:f=w1562:dbl)
            n677 = while {
              shift-right: [w1575] -> _
              shift-left: _ -> [w1570]
              shift-right: [w1572] -> _
              shift-left: _ -> [w1574]
              tunnel: w1565 -> [w1569]
              tunnel: w1562 -> [w1568]
              tunnel: w1561 -> [w1567]
              tunnel: w1559 -> [w1566]
              stop <- TRUE stop-if-true
              n678 = Get Date/Time In Seconds() -> (seconds since 1Jan1904=w1577:timestamp)
              n679 = To Double Precision Float(number=w1577) -> (double precision float=w1571:dbl)
              n680 = Build Array (concatenate)(w1574, w1568) -> (w1573:dbl[])
              n681 = case shown="\"Aero_Tunnel\"" w1569 {
                tunnel: [w1590 w1614] -> w1575
                tunnel: w1571 -> [w1589 w1614]
                tunnel: w1573 -> [w1588 w1615]
                tunnel: w1567 -> [w1587 w1613]
                tunnel: [w1586 w1615] -> w1572
                tunnel: w1568 -> [w1585 w1612]
                tunnel: w1571 -> [w1583 _]
                tunnel: w1570 -> [w1582 _]
                tunnel: w1566 -> [w1579 w1608]
                frame "Enflo_Tunnel", Default {
                  n682 = Subtract(x=w1583, y=w1582) -> (x-y=w1581:dbl)
                  n683 = Greater?(x=w1581, y=180.0) -> (0:w1580:bool)
                  n684 = And(x=w1580, y=w1579) -> (x .and. y?=w1578:bool)
                  n685 = case shown="True" w1578 {
                    tunnel: [w1592 w1605] -> w1590
                    tunnel: w1589 -> [_ w1605]
                    tunnel: w1582 -> [w1592 _]
                    tunnel: w1588 -> [w1591 w1597]
                    tunnel: w1587 -> [_ w1601]
                    tunnel: w1585 -> [_ w1594]
                    tunnel: [w1591 dbl[] []] -> w1586
                    tunnel: w1581 -> [_ w1599]
                    frame False {
                    }
                    frame True {
                      w1603 = 10.0  # In range %
                      n686 = call "Mean_fr_NaN_data.vi"("Data"=w1597) -> ("Mean value"=w1595:dbl)  [unwired: 1 out]
                      n687 = Less?(x=w1599, y=60.0) -> (x < y?=w1596:bool)
                      n688 = Select(t=w1595, s=w1596, f=w1594) -> (s? t:f=w1593:dbl)
                      n689 = call "Hydrosonic_Conrol.vi"("In range %"=w1603, "Input Mode"=enum16{"Desired Frequency", "Transducer value"}."Desired Frequency", "Actual Sampling rate (Hz)"=w1593, "Desired Value"=w1601) -> ("Set output"=w1602:dbl)  [unwired: 1 out]
                      n690 = call "Display_LDA_data_rate.vi"("Hydrosonic Setting %"=w1602, "Current Sampling Freq (Hz)"=w1594) -> ()  [unwired: 1 out]
                    }
                  }
                }
                frame "Aero_Tunnel" {
                  n691 = call "Get_Current_Scan_client.vi"("singleChannel"="Aero_Tunnel:Motor:Enable" ("Channel Name")) -> ("Numerical Values"=w1611:dbl[])  [unwired: 1 in, 3 out]
                  n692 = Index Array(array=w1611) -> (element=w1610:dbl)  [unwired: 1 in]
                  n693 = Greater Than 0?(x=w1610) -> (x > 0?=w1609:bool)
                  n694 = And(x=w1609, y=w1608) -> (x .and. y?=w1607:bool)
                  n695 = case shown="True" w1607 {
                    tunnel: w1613 -> [_ w1624]
                    tunnel: w1612 -> [w1616 w1621]
                    frame False {
                      # "Control Seeder Manually"
                      n696 = call "Display_LDA_data_rate.vi"("Current Sampling Freq (Hz)"=w1616) -> ()  [unwired: 1 in, 1 out]
                    }
                    frame True {
                      n697 = Multiply(x=1.05, y=w1624) -> (x*y=w1623:dbl)
                      n698 = Greater Or Equal?(x=w1621, y=w1623) -> (x >= y?=w1627:bool)
                      n699 = Select(t=0.0, s=w1627, f=1.0) -> (s? t:f=w1618:dbl)
                      n700 = call "Display_LDA_data_rate.vi"("Hydrosonic Setting %"=w1618, "Current Sampling Freq (Hz)"=w1621) -> ()  [unwired: 1 out]
                      n701 = Build Array("Aero_Tunnel:Seeder:Enable" ("Channel Name")) -> (w1619:string[])
                      n702 = Build Array(w1618) -> (w1617:dbl[])
                      n703 = call "ASYNC_Adam_client.vi"("Values"=w1617, "Channel Names"=w1619) -> ()  [unwired: 1 in, 2 out]
                    }
                  }
                }
              }
            }
          }
        }
      }
    }
  }
